vi "DB - [Execute].[Transaction].vi"(0 "connection reference":T12, 1 "DB.Schema.Table":string="SRTRS.Execute.TransactionResult", 2 "DB.Schema.Table 2\n(NA)":string, 3 "String ([RawDataFile] Filestream)":string, 4 "Transaction":T4, 5 "error in (no error)":errorcluster, 6 "DB Connection":T8={"Open"=TRUE, "Close"=TRUE}, 7 "Refnums":T7, 8 "DB - Execute Transaction":T6, 9 "[RawDataFileName]":string, 10 "[TransactionResult] v02":T5[](array[typedef]), 11 "DB Refnums II":T2, 12 "<Values>":string[](array[string])) -> (14 "connection reference":T12, 16 "1D Results":string[](array[string]), 18 "Transaction":T4, 19 "SUMMARY":errorcluster)   [LabVIEW 2013]
uses:
  <vilib>/addons/database/Connection.llb/Conn ObjectReference.ctl
  Controls/Setup - Part Details - Item Details.ctl
  Controls/Combo Box.ctl
  Controls/DB - Logon Info.ctl
  Controls/DB - OpenClose.ctl
  Controls/DB - Refnums.ctl
  Controls/DB - Execute Transaction Enum.ctl
  Controls/DB - [TransactionResult] Enum.ctl
  Controls/Transaction Cluster.ctl
  Controls/DB - Refnums II.ctl
  Controls/Execute - Info.ctl
  Controls/DB - [Execute].[Header] ColNames.ctl
  Controls/Global SRTRS.vi
  <vilib>/addons/database/Connection.llb/DB Tools Open Connec (String).vi
  <vilib>/addons/database/Connection.llb/Conn Execute.vi
  <vilib>/addons/database/Recordset.llb/Rec Fetch String Data (R).vi
  <vilib>/addons/database/Recordset.llb/Rec Destroy - Connection.vi
  <vilib>/addons/database/Recordset.llb/Rec Fetch Recordset Data (R).vi
  <vilib>/addons/database/NI_Database_API.lvlib
panel:
  in  "Equipment Details":i32(listbox)=-1
  in  "Info. (Execute Tab)":T1 caption="Info." {"Variant Allowed (Hold Temp)" format="%.1f"}
  in  "Results Output":cluster{"Output Set":T3, "Description":string}
  out "Close error out":errorcluster
  in  "MCListBox FHS Setup":i32(listbox)=-1 caption="Furnace Heating Sequence"
  out "Refnums error out":errorcluster={"status"=TRUE, "code"=1055, "source"="To More Specific Class in DB - Setup Item (Part Details).vi->Main.vi"}
  in  "Part Details":i32(listbox)=-1
  in  "MCListBox AWPS":i32(listbox)=-1 caption="Additional WPS/Ref MCListBox"
  in  "Logon":T9={"PlantID"="4070", "SystemID"="SRSB-2A", "UserID"="100001", "DomainID"="CCC", "LanguageID"="EN", "StationID"=""}
  in  "WPS Details Setup":T10={"WPS/Ref"="WPS5", "Rev"="1", "Hold Temperature"="100", "WPS Details Temperature Units"="°C", "Hold Time (HH:MM)"="1:00", "Inactive"=FALSE} caption="WPS Details"
  in  "Extra WPS":string caption="WPS"
  in  "Extra Rev":string caption="Rev."
  out "SQL 1":string
  in  "Item Details":T11={"Order No."="102", "Oper. No."="102", "Qty."=1, "NCR No."="102", "NCR Boolean"=FALSE, "Customer No."="102", "Customer Name"="Cust102", "Project"="Proj102", "Sales Order"="SO102", "Item No."="SOI102", "Material"="M102", "Revision"="1", "Material Description"="", "Serial No."="102", "UnitOfQty"="Pallet"} {"Qty." min=1 max=99}
  in  "Notes":string="Hello World"
  out "ms":u32
  out "SQL 2":string="USE [SRTRS]\n\nIF EXISTS(SELECT 1 from [Config].[Mapping]\nwhere [TransactionNo] = '<A>' )\n\nBEGIN\nDELETE FROM [MasterData].[Material]\nWHERE  [TransactionNo] = '<A>' \nEND\n\nINSERT INTO [Config].[Mapping]\n           ([TransactionNo]\n           ,[ItemNo]\n           ,[OrderNo]\n           ,[OperationNo]\n           ,[Qty]\n           ,[UnitOfQty]\n           ,[NCRIndicator]\n           ,[NCRNo]\n           ,[CustomerID]\n           ,[Customer]\n           ,[Project]\n           ,[SalesOrderNo]\n           ,[SalesOrderItemNo]\n           ,[MaterialNo]\n           ,[MaterialDesc]\n           ,[MaterialRev]\n           ,[SerialNos]\n           ,[Notes]\n           ,[TC01]  ,[TC02]  ,[TC03] ,[TC04] ,[TC05] ,[TC06] \n           ,[TC01Plot] ,[TC02Plot] ,[TC03Plot] ,[TC04Plot] ,[TC05Plot] ,[TC06Plot] \n           )\nVALUES (('' ,'1' ,'SOI101' ,'101' ,'101' ,'1' ,'EA' ,'FALSE' ,'101' ,'101' ,'Cust101' ,'Proj101' ,'SO101' ,'SOI101' ,'M101' ,'MD101' ,'1' ,'101' ,'' ,'1' ,'' ,'' ,'' ,'' ,'' ,'' ,'' ,'' ,'' ,'' ,'' ),('' ,'2' ,'SOI102' ,'102' ,'102' ,'1' ,'Pallet' ,'FALSE' ,'102' ,'102' ,'Cust102' ,'Proj102' ,'SO102' ,'SOI102' ,'M102' ,'2' ,'1' ,'102' ,'' ,'2' ,'' ,'' ,'' ,'' ,'' ,'' ,'' ,'' ,'' ,'' ,'' ))\n\n-- SELECT SCOPE_IDENTITY()"
  out "Connection Information":T13={"Connection "="SQL Server 32bit HPEnvy", "Username"="admin", "Password"="admin123"}
  # "Column Hdrs[] are Important \nMust match with SRTRS Main.vi"
  # "Min"
  # "Min"
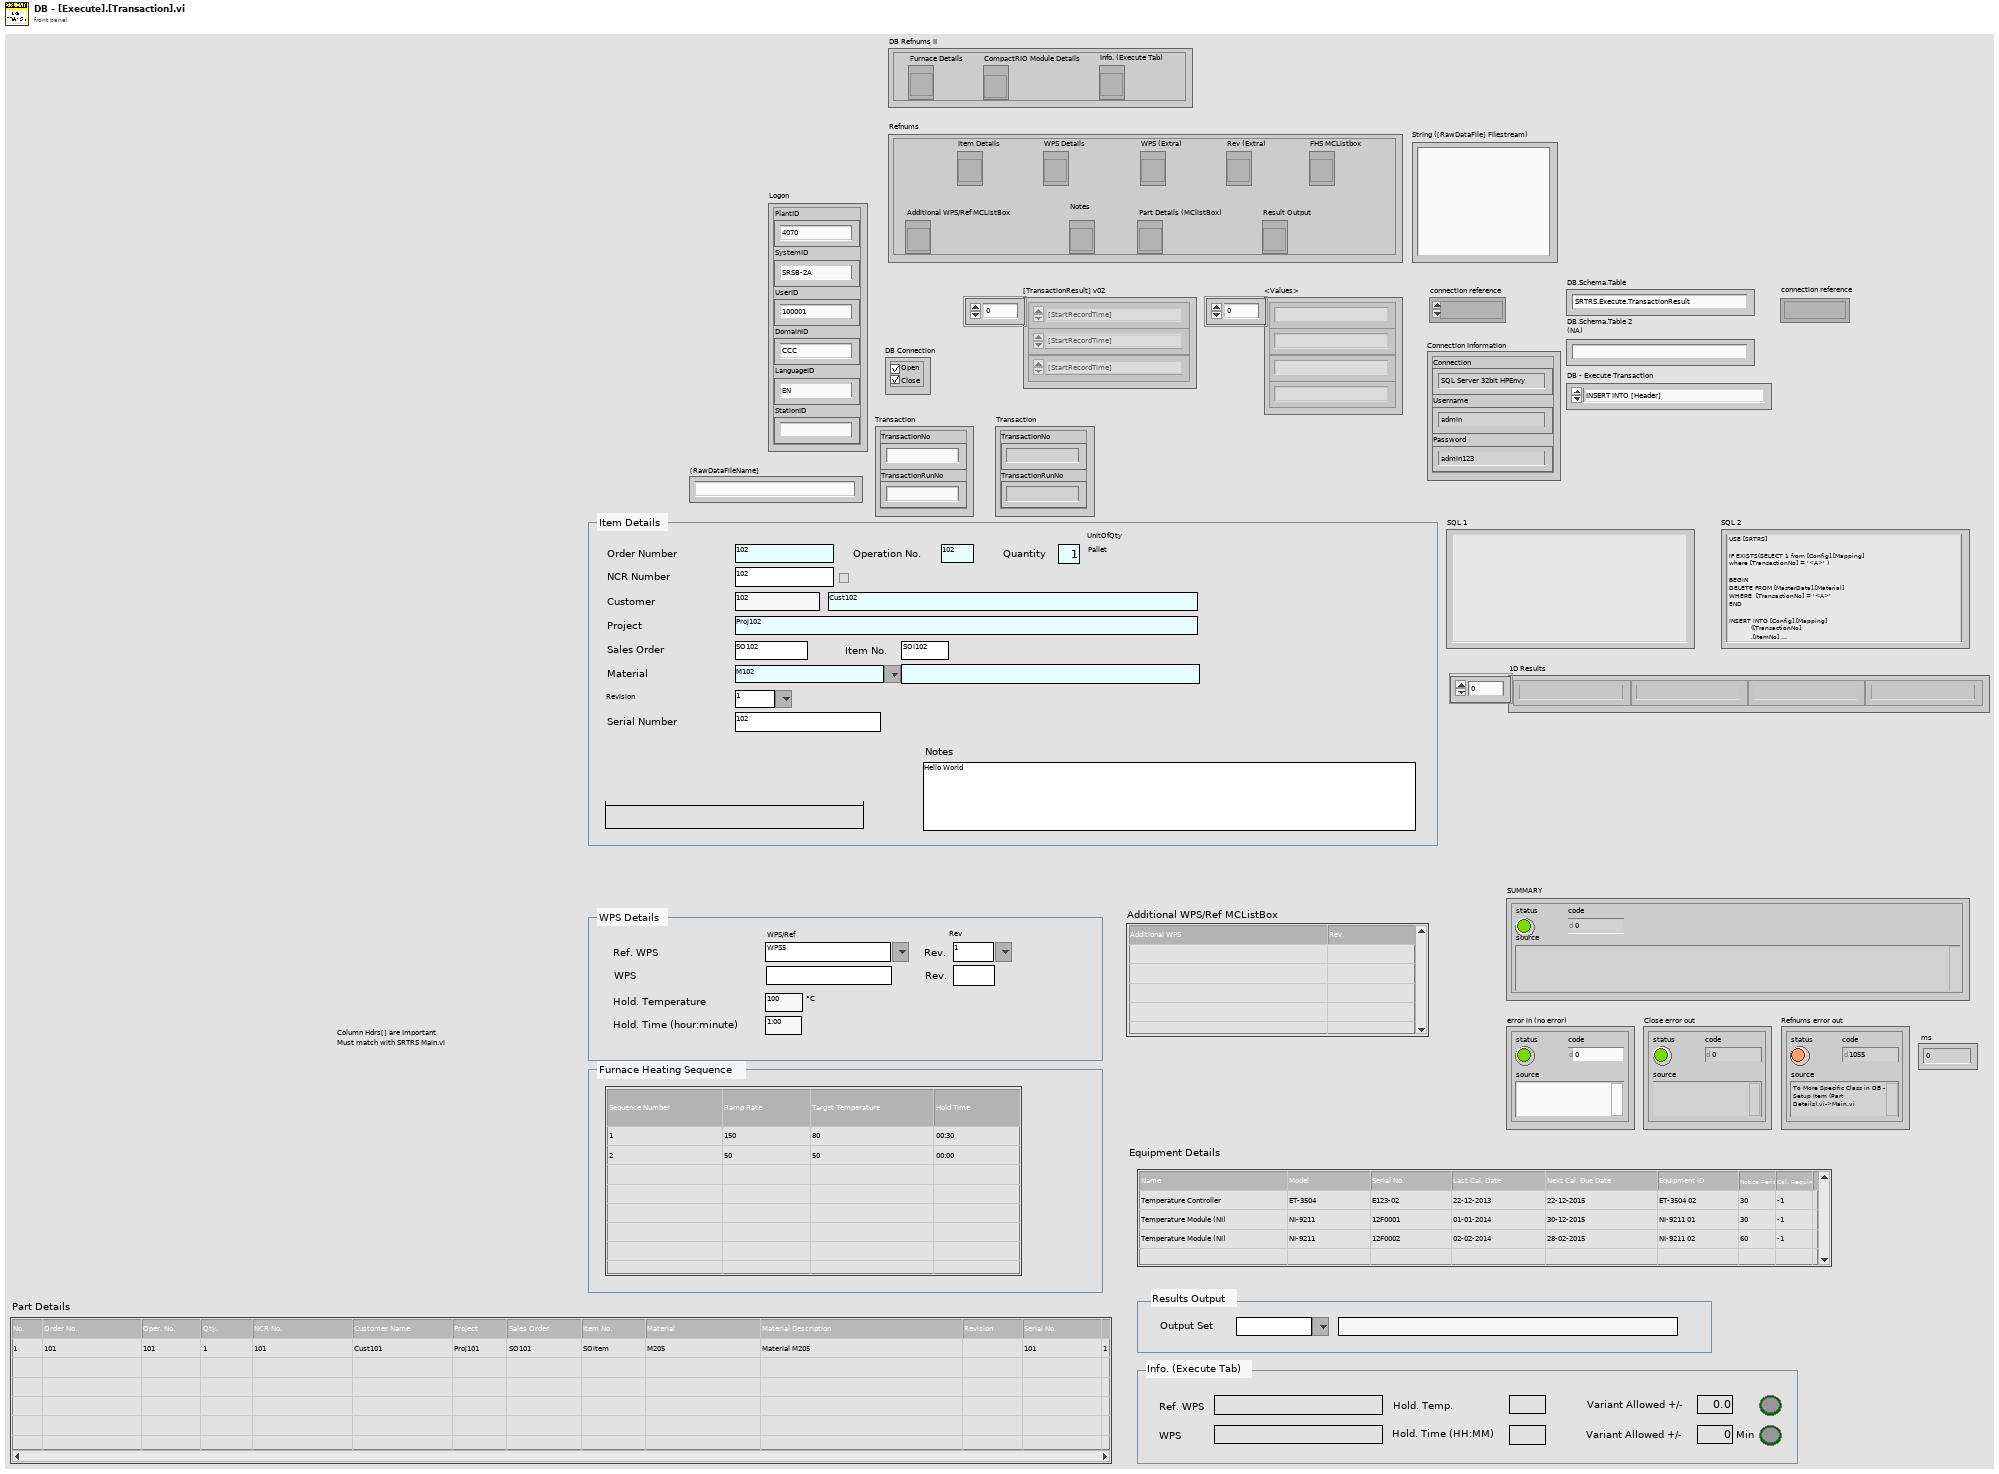
[diagram p1: front panel]
types:
  T1 = typedef "Execute - Info.ctl" = cluster{"Ref WPS":string, "Hold. Temp.":string, "Info. Temperature Units":string, "Variant Allowed (Hold Temp)":dbl, "Info. Temperature Units 2":string, "Variant Allowed (Hold Temp)":bool, "Hold. Time (hour:minute)":string, "Variant Allowed (Hold Time)":dbl, "Variant Allowed (Hold Time)":bool, "WPS":string}
  T2 = typedef "DB - Refnums II.ctl" = cluster{"Furnace Details":refnum<vi>, "CompactRIO Module Details":refnum<vi>, "Info. (Execute Tab)":refnum<vi>}
  T3 = typedef "Combo Box.ctl" = string
  T4 = typedef "Transaction Cluster.ctl" = cluster{"TransactionNo":string, "TransactionRunNo":string}
  T5 = typedef "DB - [TransactionResult] Enum.ctl" = enum16{"[StartRecordTime]", "[StartRecordTemp]", "[MaxRecordedTemp]", "[MaxRecordedTempTime]", "[MinRecordedTemp]", "[MinRecordedTempTime]", "[EndRecordTemp]", "[EndRecordTime]", "[RecordedMinutes]", "[StartHoldTime]", "[StartHoldTemp]", "[HoldTimeMaxTemp]", "[HoldTimeMaxTempTime]", "[HoldTimeMinTemp]", "[HoldTimeMinTempTime]", "[EndHoldTime]", "[EndHoldTemp]", "[HoldDurationMinutes]", "[TempDiffDuringHold]", "[UnitOfTemperature]", "[PerformedBy]", "[PerformedOn]", "[IsTempWithinTol]", "[IsTimeWithinTol]", "[HoldTimePercentage]", "[ProcessStatus]", "[OverallStatus]", "[SequenceStatus]", "[Parameter1]", "[Parameter2]", "[Parameter3]", "[Parameter4]", "[Parameter5]", "[Parameter6]", "[Parameter7]", "[Parameter8]", "[Parameter9]", "[Parameter10]", "[Parameter11]", "[Parameter12]", "[Result]", "[RawDataFile]", "[RawDataFilePath]", "[RawDataFileName]", "[OutputSetId]", "[SavedBy]", "[SavedOn]", "[Inactive]"}
  T6 = typedef "DB - Execute Transaction Enum.ctl" = enum16{"INSERT INTO [Header]", "INSERT INTO [TransactionResult]", "INSERT INTO [ProcedureItem]", "INSERT/UPDATE [Execute].[Active]", "SELECT [Execute].[Active]", "UPDATE [TransactionResult]", "UPDATE FILESTREAM", "SELECT [TransactionResult]", "SELECT [TransactionNo],[TransactionRunNo]"}
  T7 = typedef "DB - Refnums.ctl" = cluster{"Item Details":refnum<vi>, "WPS Details":refnum<vi>, "WPS (Extra)":refnum<vi>, "Rev (Extra) ":refnum<vi>, "FHS MCListbox":refnum<vi>, "Additional WPS/Ref MCListBox":refnum<vi>, "Notes":refnum<vi>, "Part Details (MClistBox)":refnum<vi>, "Result Output":refnum<vi>}
  T8 = typedef "DB - OpenClose.ctl" = cluster{"Open":bool, "Close":bool}
  T9 = typedef "DB - Logon Info.ctl" = cluster{"PlantID":string, "SystemID":string, "UserID":string, "DomainID":string, "LanguageID":string, "StationID":string}
  T10 = cluster{"WPS/Ref":T3, "Rev":T3, "Hold Temperature":string, "WPS Details Temperature Units":string, "Hold Time (HH:MM)":string, "Inactive":bool}
  T11 = typedef "Setup - Part Details - Item Details.ctl" = cluster{"Order No.":string, "Oper. No.":string, "Qty.":i32, "NCR No.":string, "NCR Boolean":bool, "Customer No.":string, "Customer Name":string, "Project":string, "Sales Order":string, "Item No.":string, "Material":string, "Revision":string, "Material Description":string, "Serial No.":string, "UnitOfQty":string}
  T12 = typedef "NI_Database_API.lvlib/Conn ObjectReference.ctl" = refnum<k1>
  T13 = cluster{"Connection ":string, "Username":string, "Password":string}
  T14 = typedef "Enum - InteractiveMode-SubVIMode.ctl" = enum16{"Interactive", "subVI Mode"}
  T15 = typedef "Connection Information Cluster.ctl" = cluster{"Connection ":string, "Username":string, "Password":string}
  T16 = typedef "DB - DB.Schema.Table.ctl" = cluster{"DB":string, "Schema":string, "Table":string}
  T17 = typedef "DB - [Execute].[Header] ColNames.ctl" = enum16{"[SystemId]", "[PlantId]", "[StationId]", "[ProcedureNo]", "[ProcedureRev]", "[WpsNo]", "[WpsRev]", "[HoldTemperature]", "[UnitOfTemperature]", "[HoldTime]", "[OutputSetId]", "[AdditionalProcs]", "[Equipment1Id]", "[Equipment2Id]", "[Equipment3Id]", "[Equipment4Id]", "[Equipment5Id]", "[Equipment6Id]", "[Equipment7Id]", "[Equipment8Id]", "[Equipment9Id]", "[Equipment10Id]", "[PermittedTempDiff]", "[PermittedTimeDiff]", "[Notes]", "[LastSavedBy]", "[LastSavedOn]", "[Indicator1]", "[Indicator2]", "[Remark1]", "[Remark2]", "[Remark3]", "[Remark4]", "[Inactive]"}
  T18 = typedef "NI_Database_API.lvlib/Rec ObjectReference.ctl" = refnum<k1>
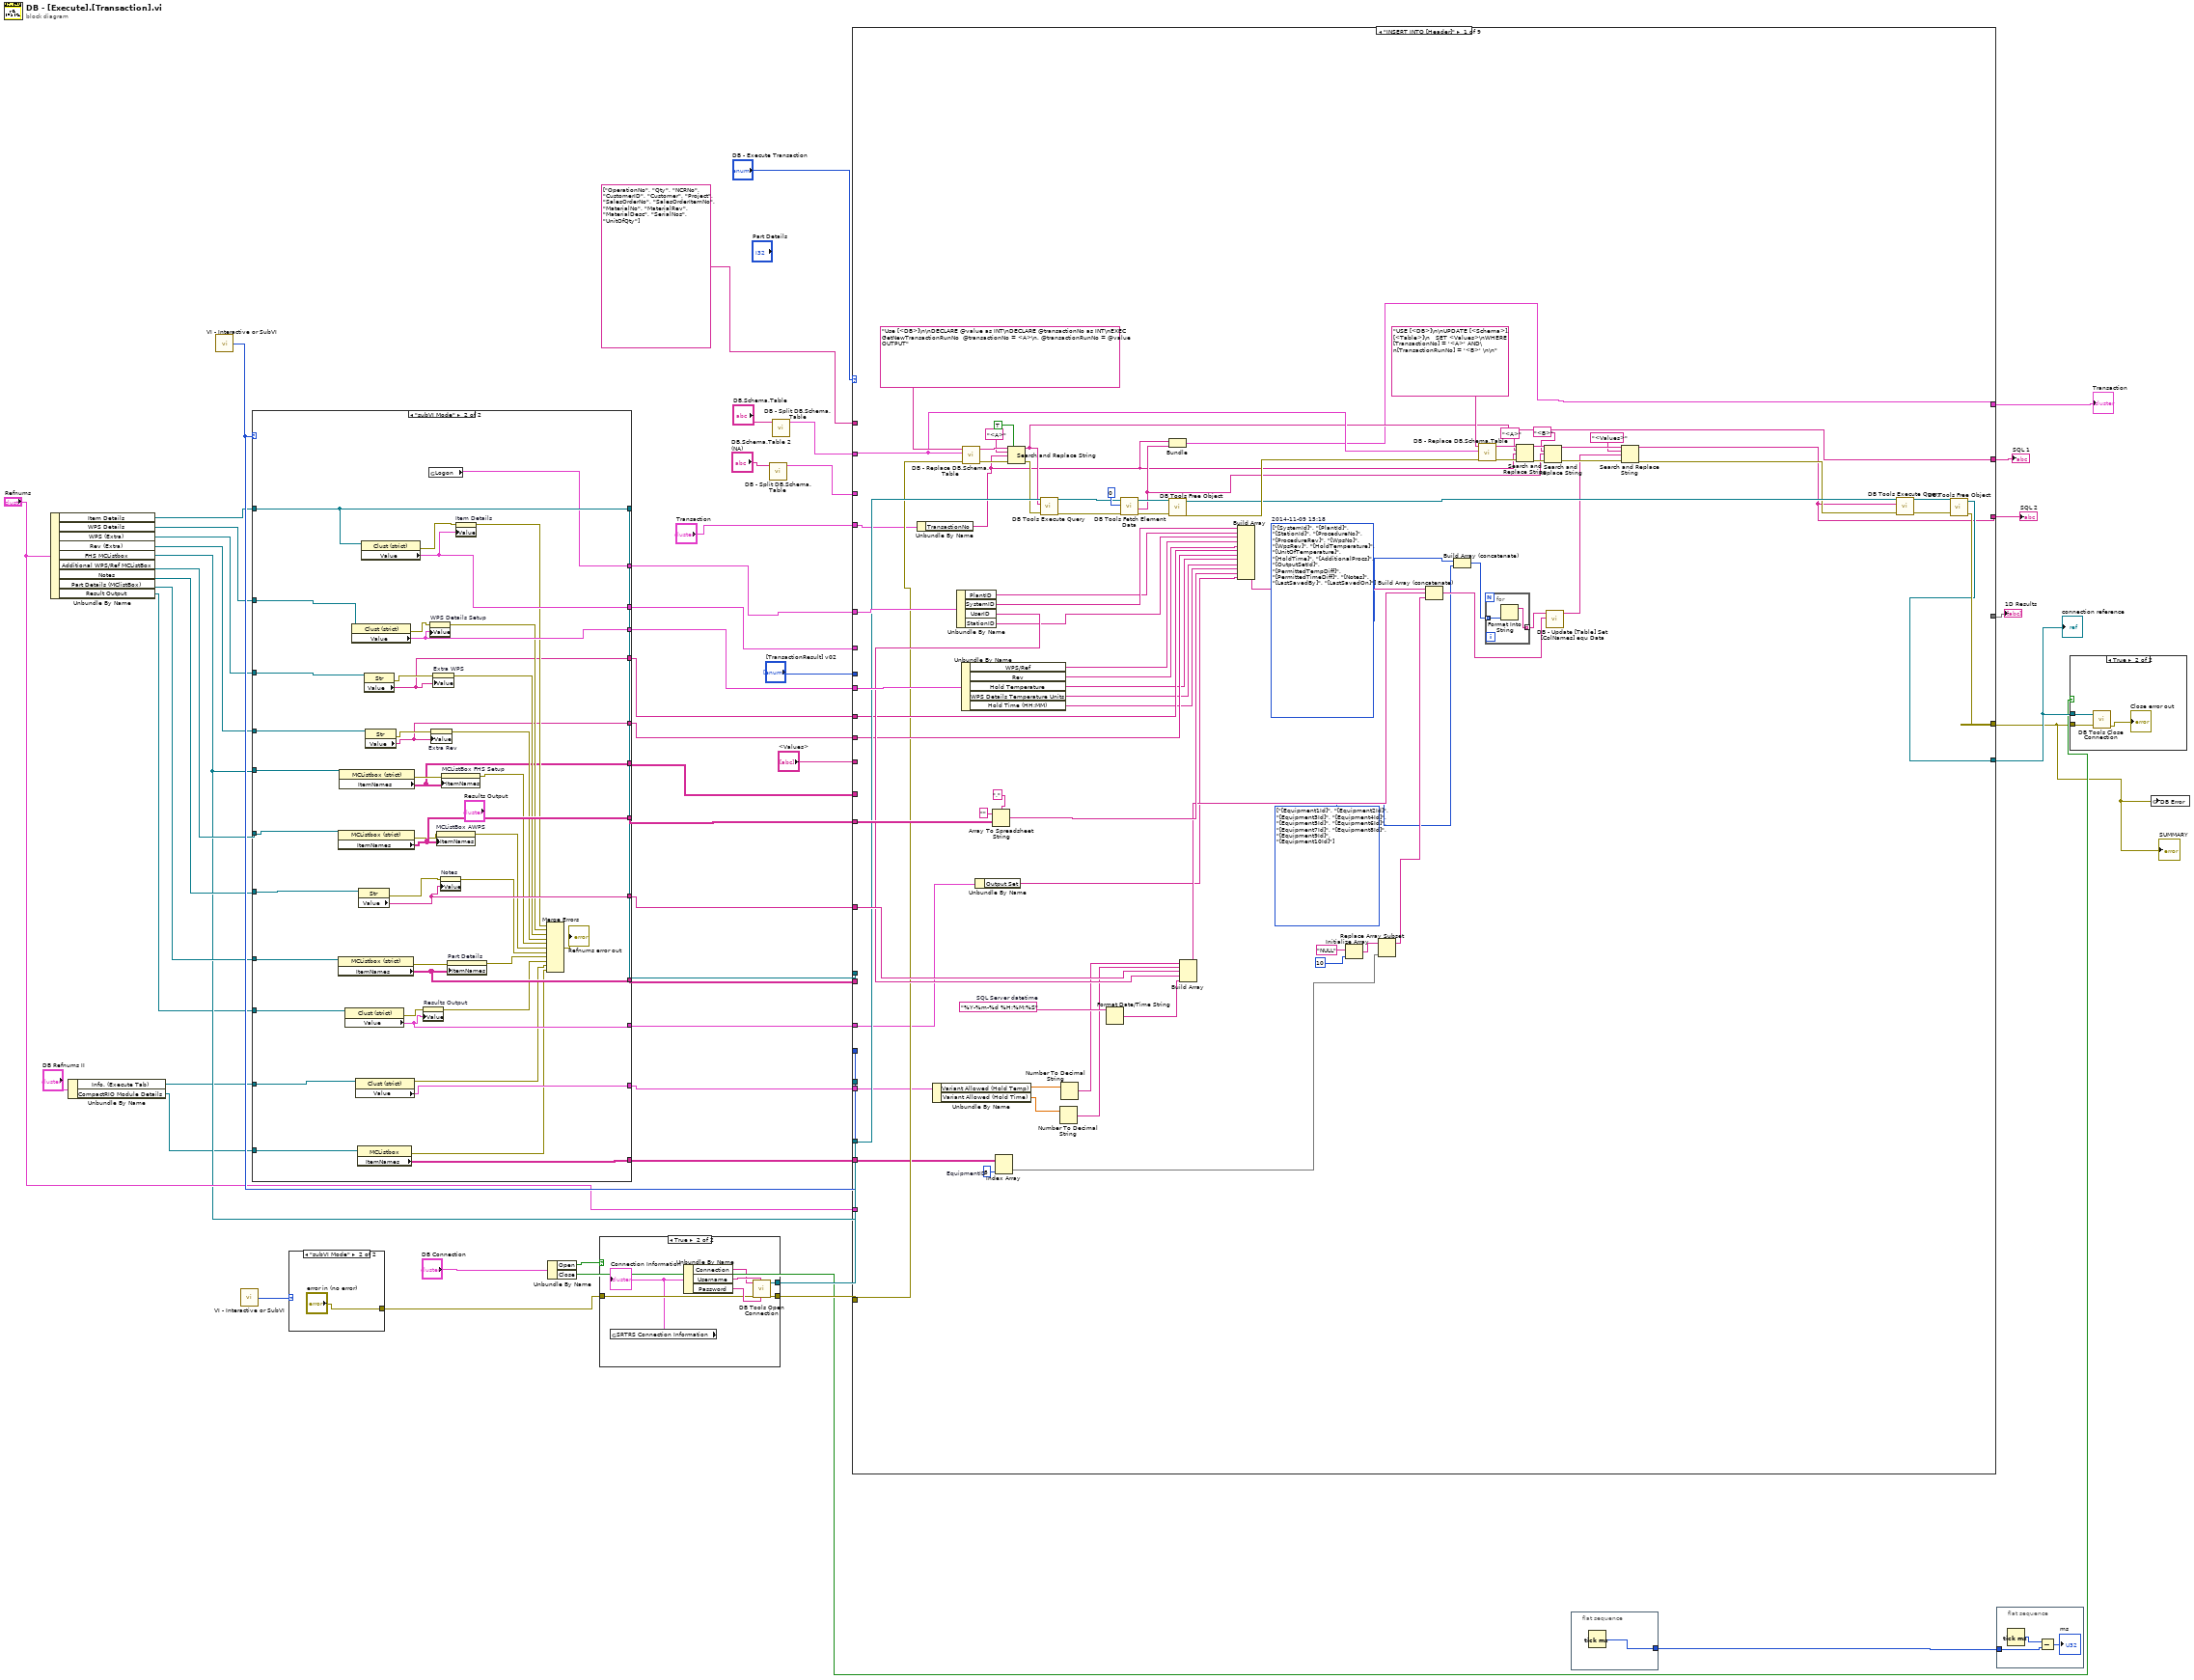
[diagram p0: block diagram]
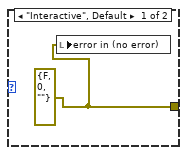
[diagram p2: hidden frame]
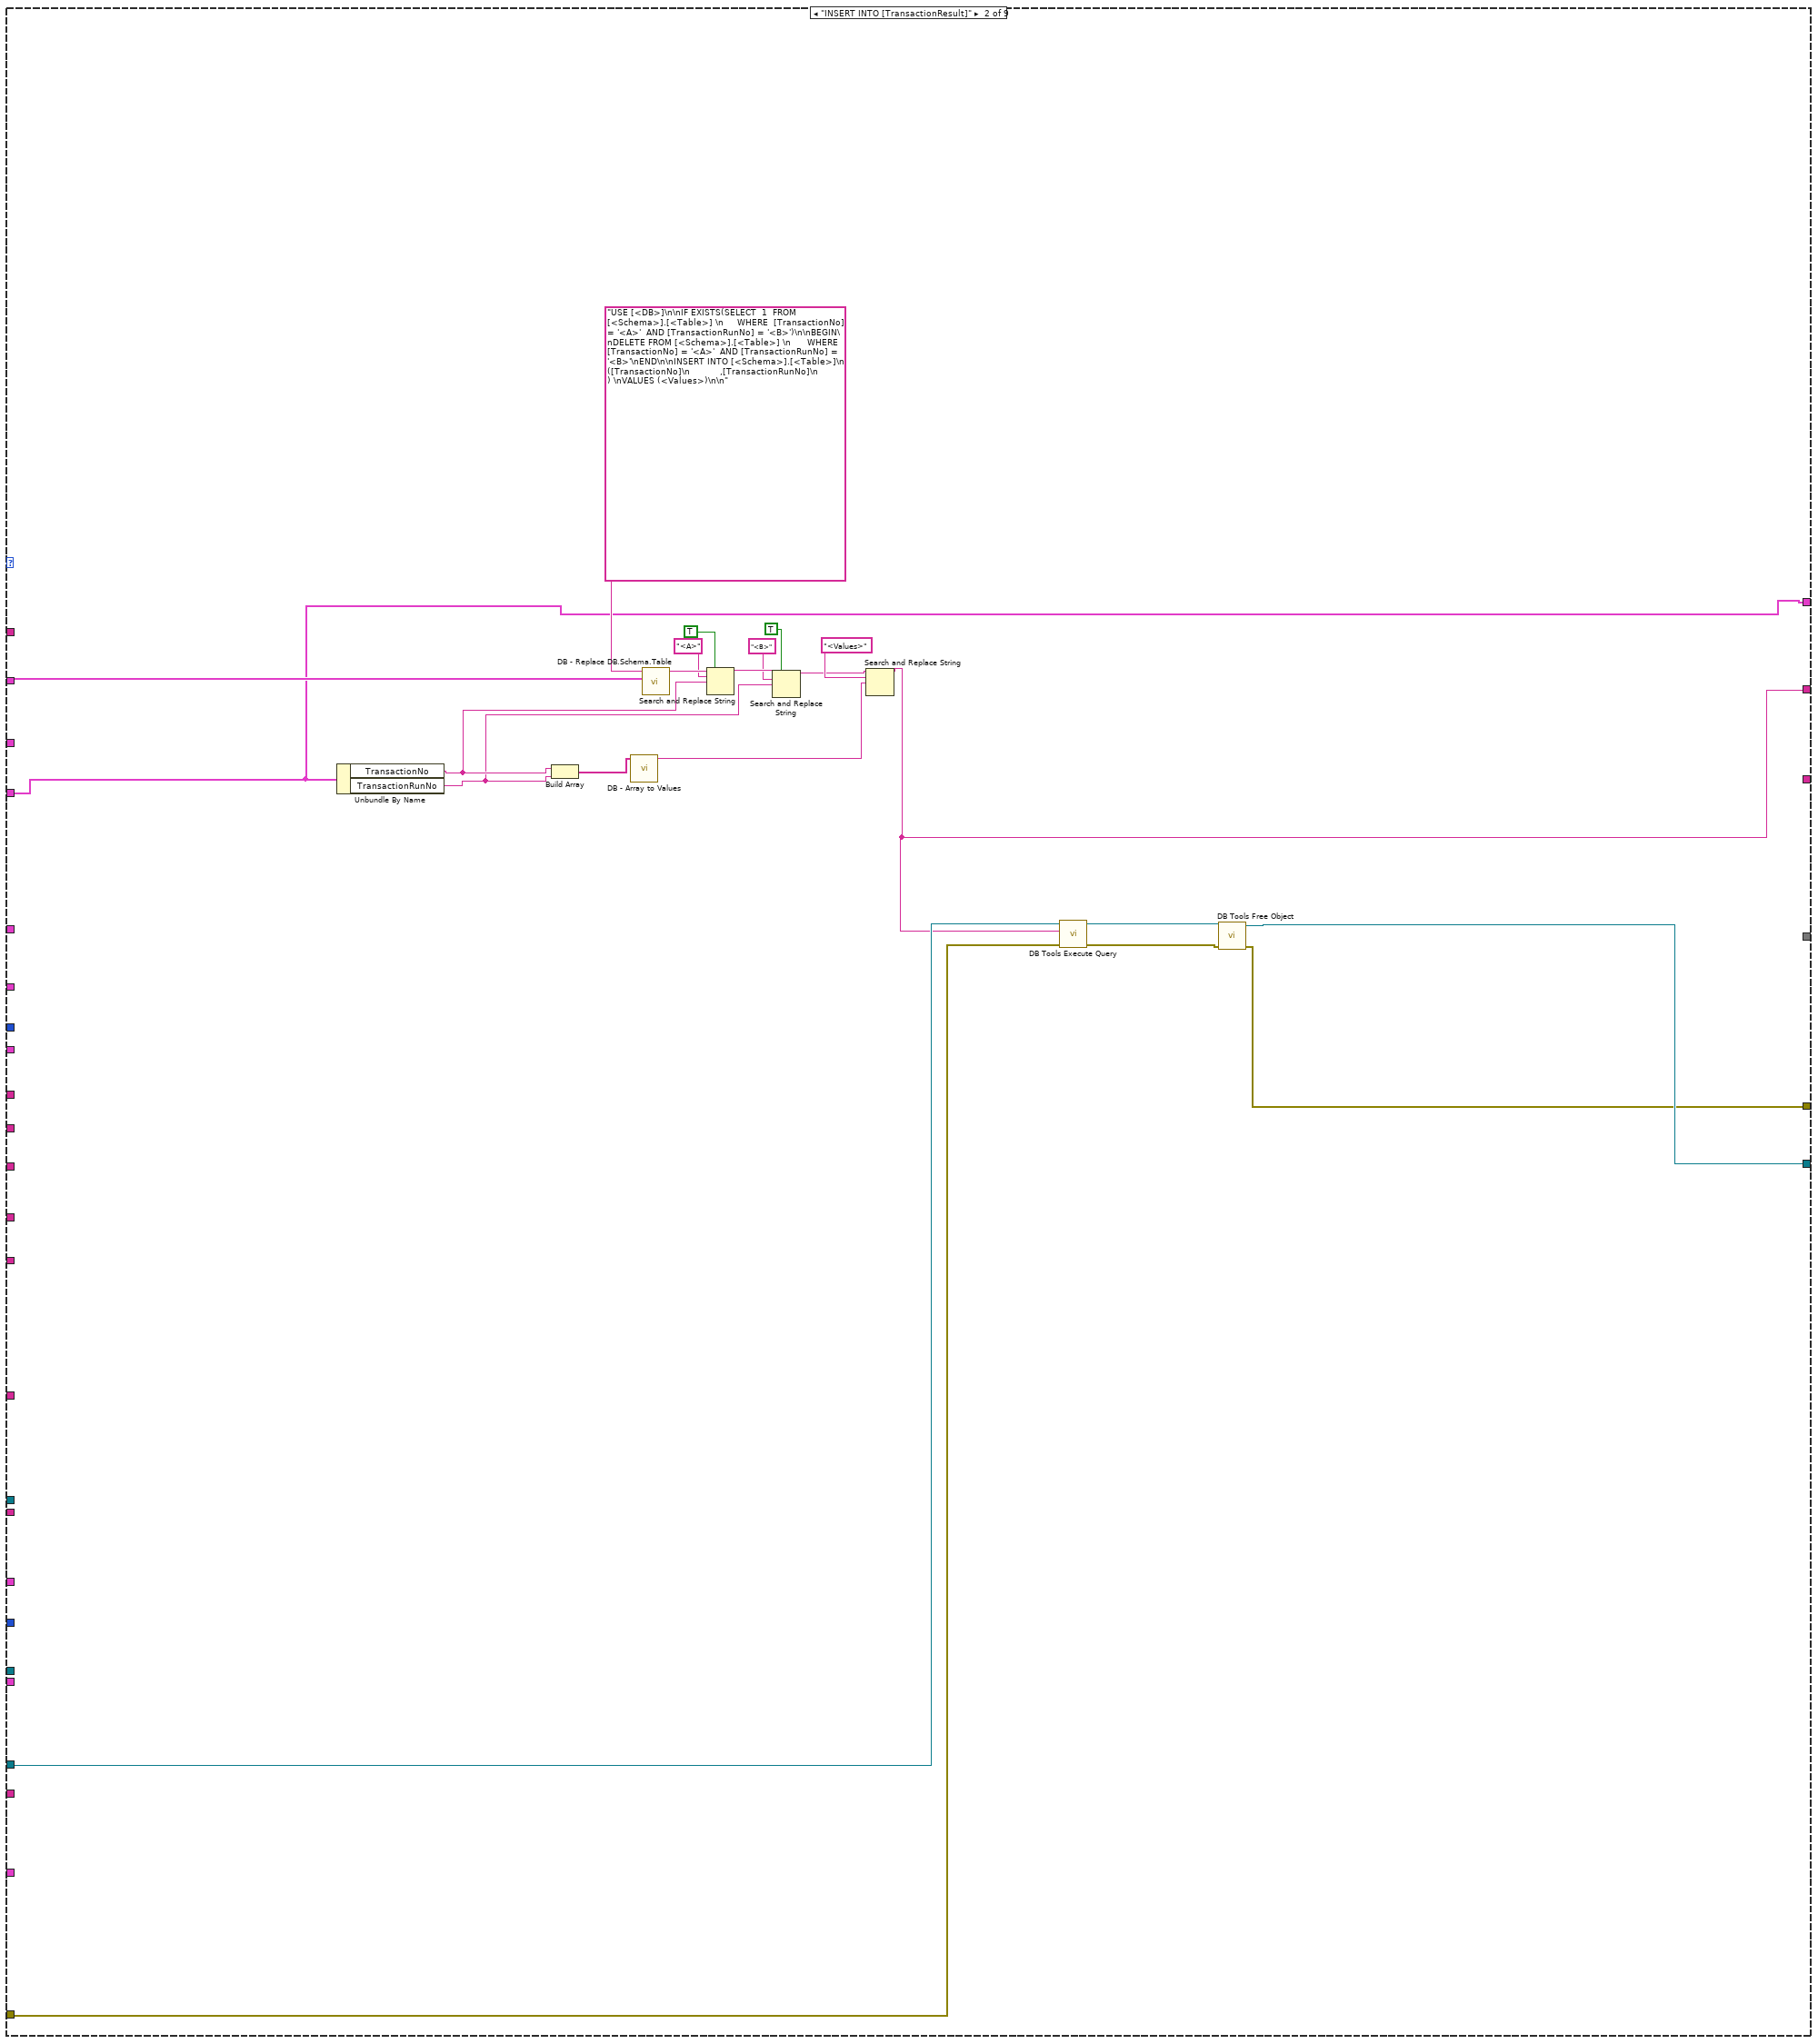
[diagram p3: hidden frame]
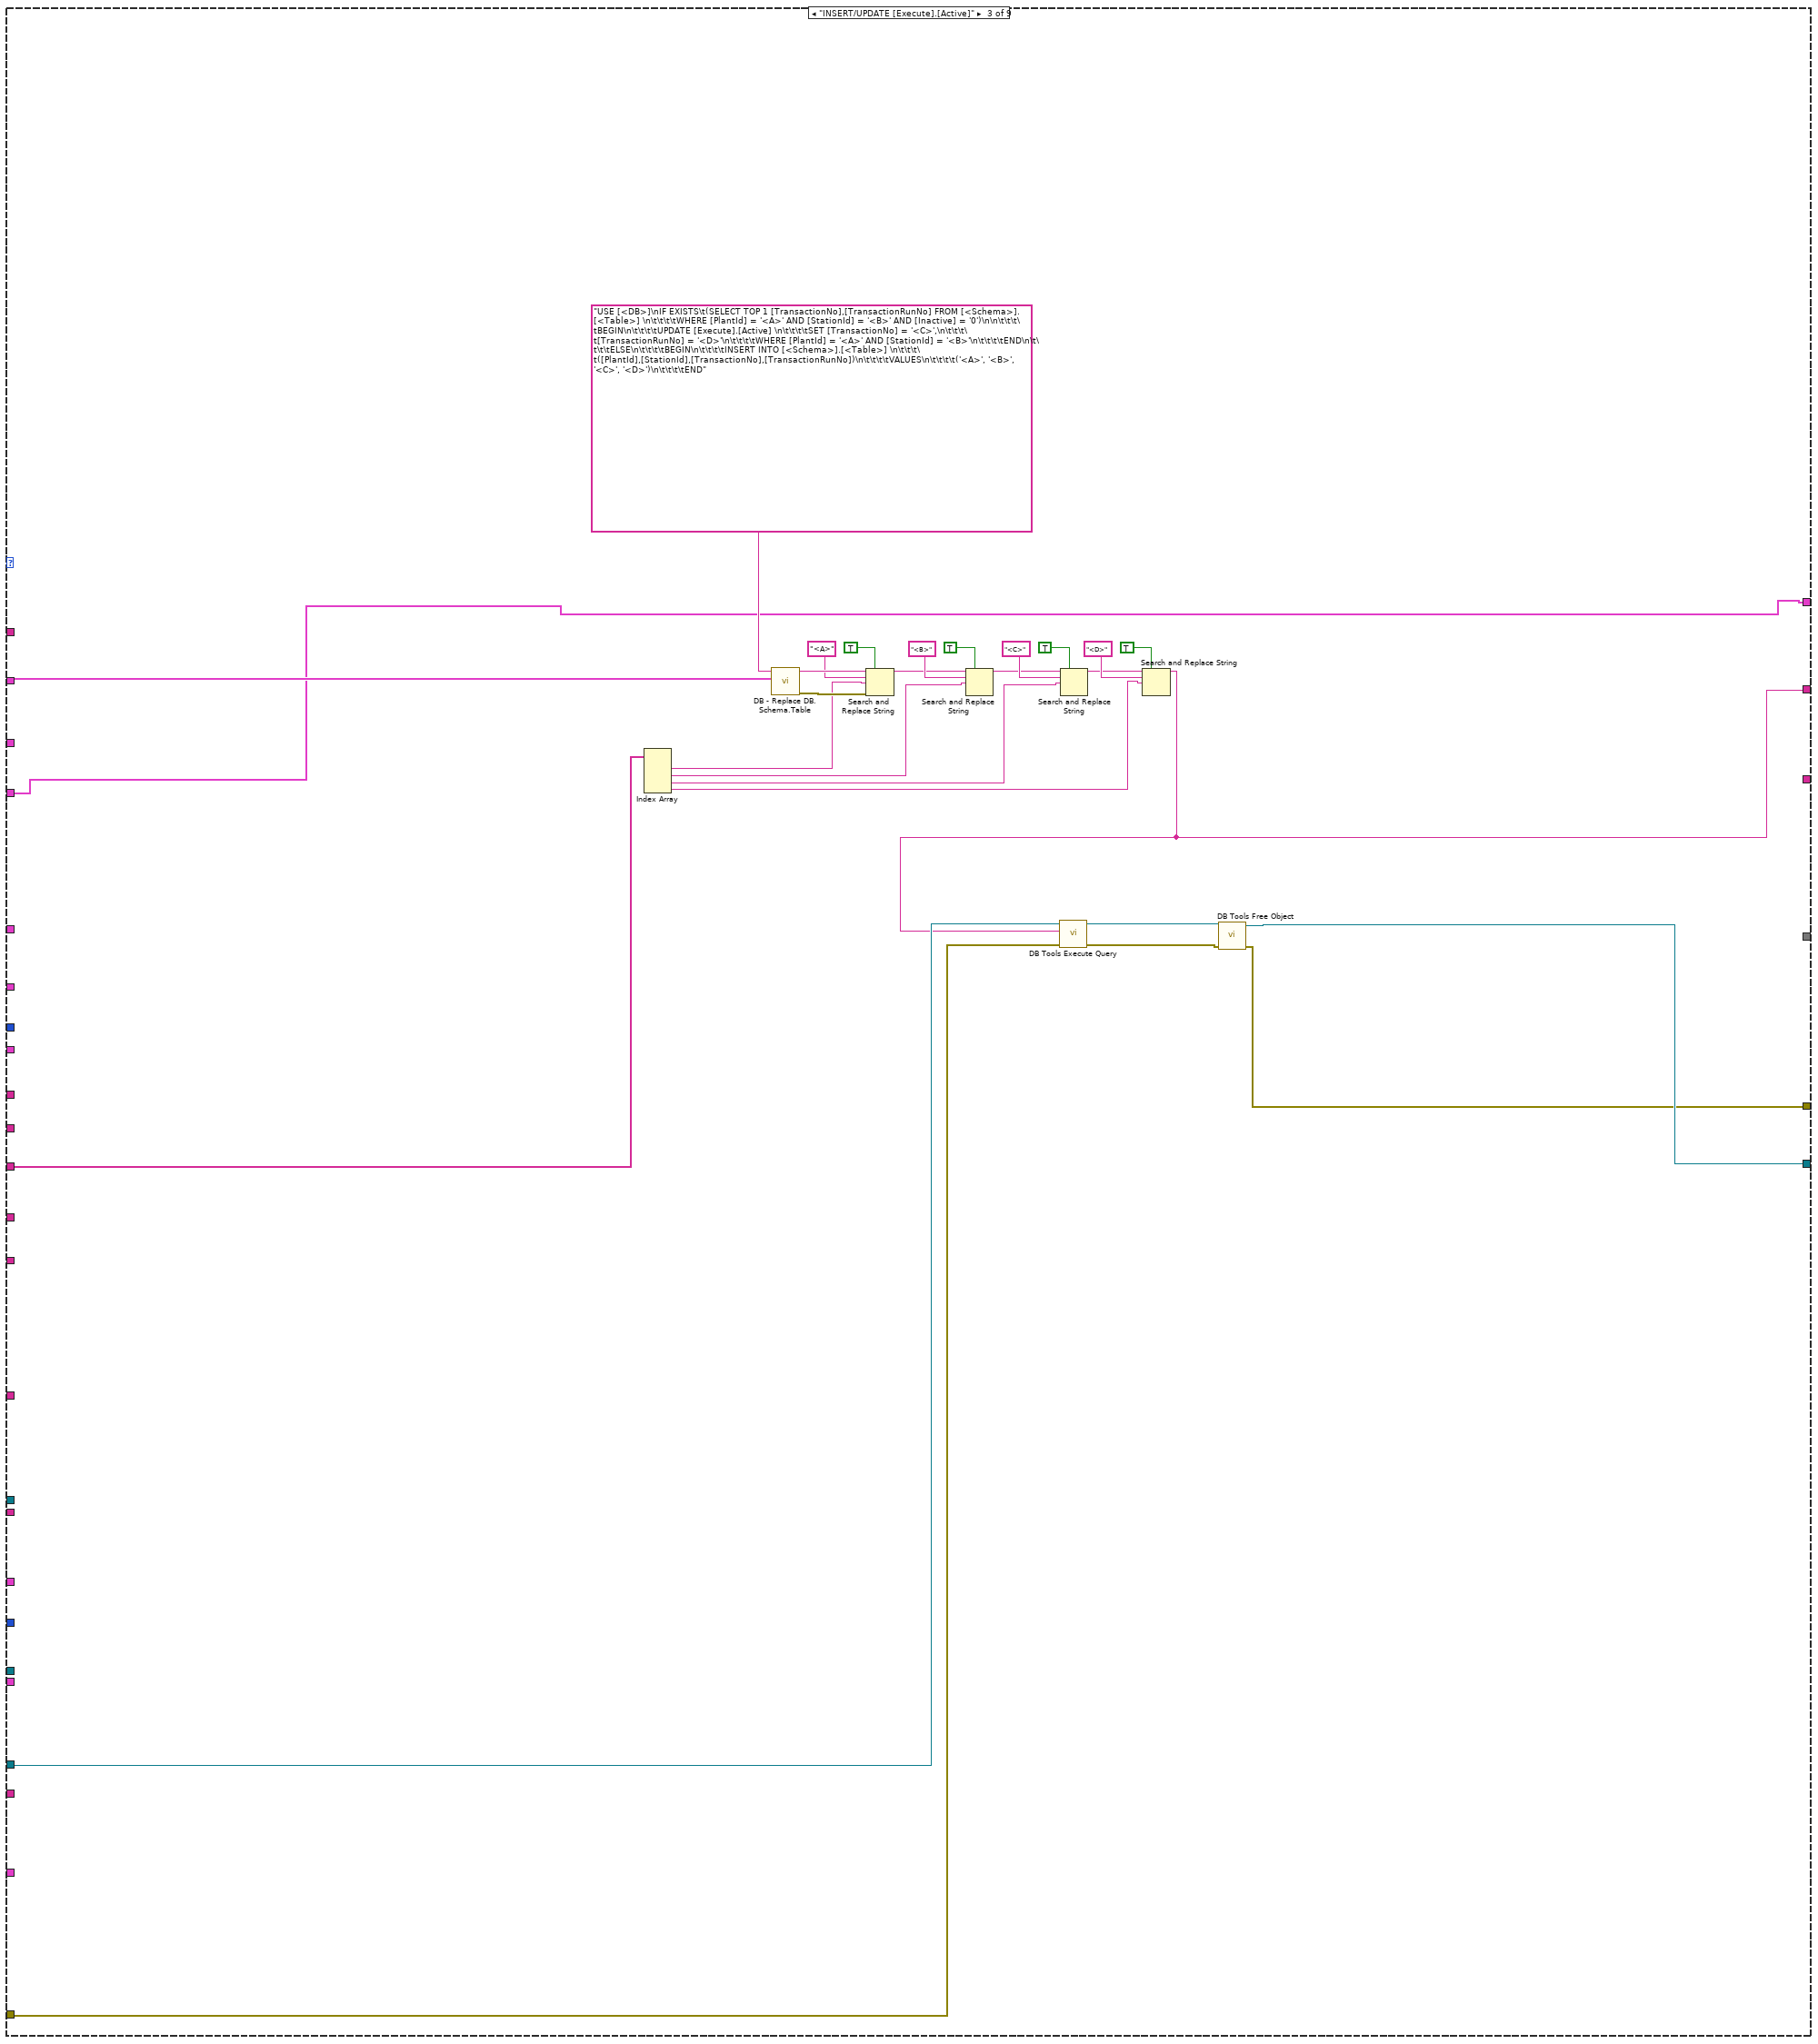
[diagram p4: hidden frame]
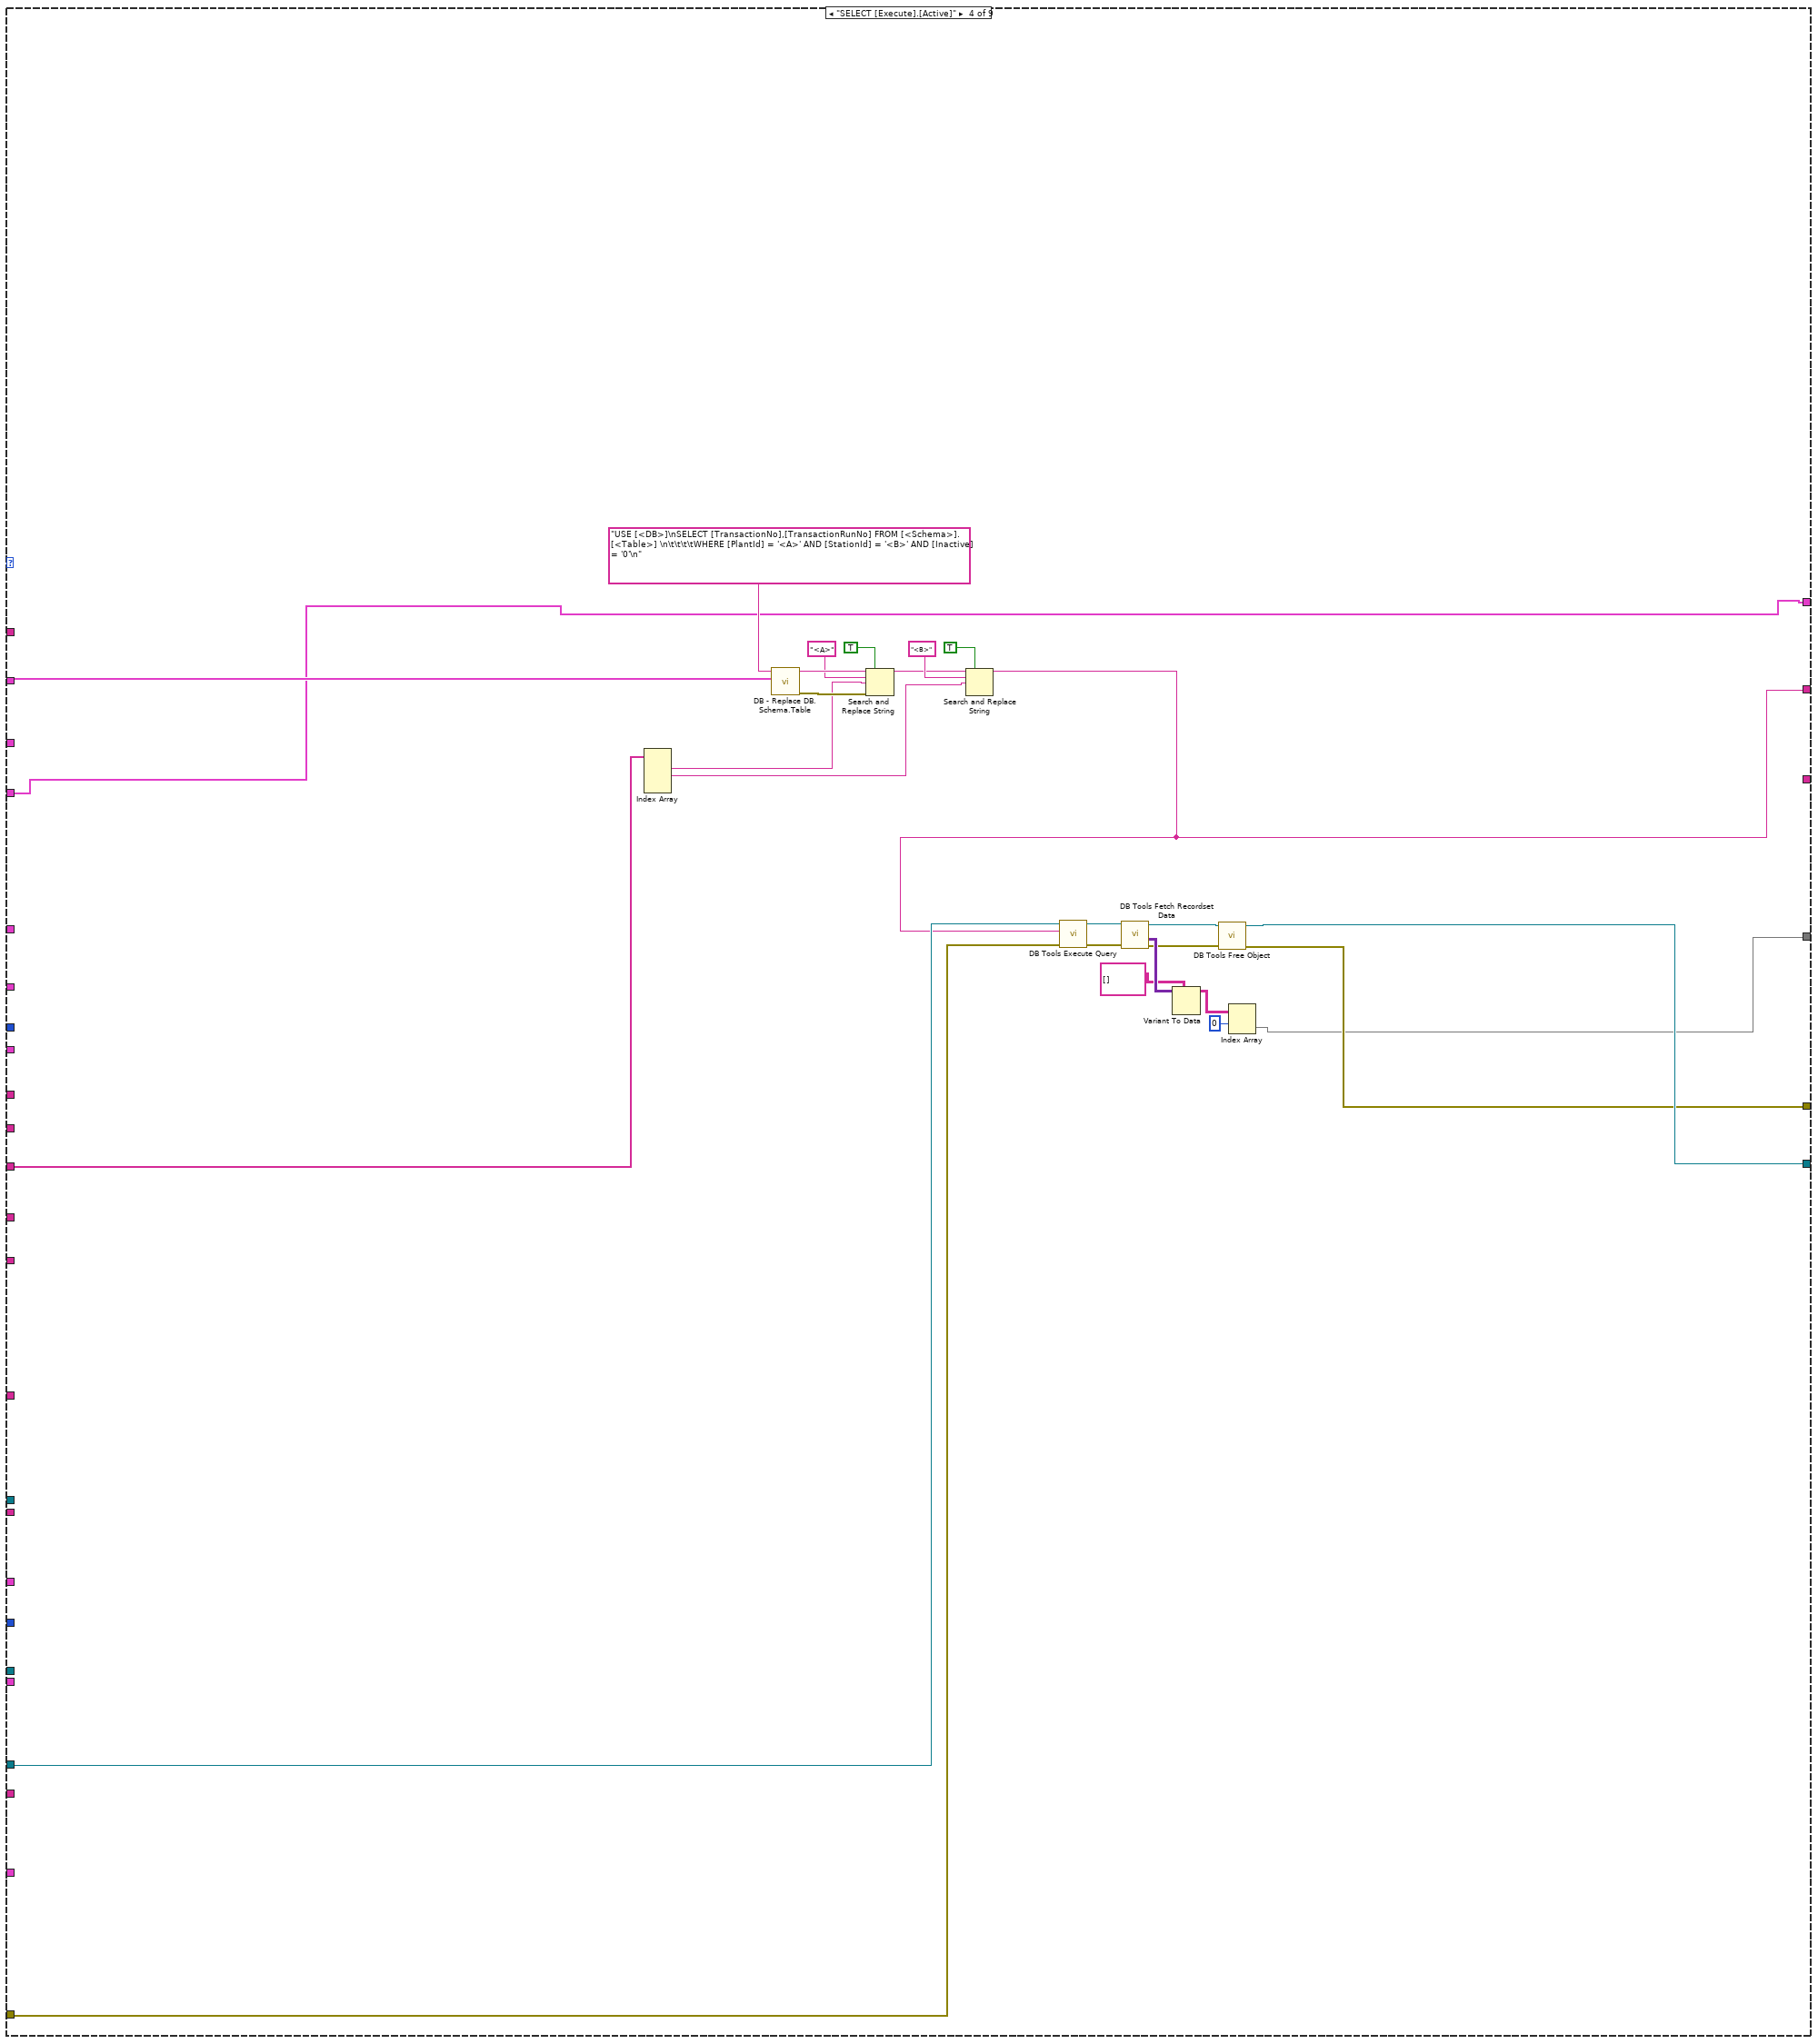
[diagram p5: hidden frame]
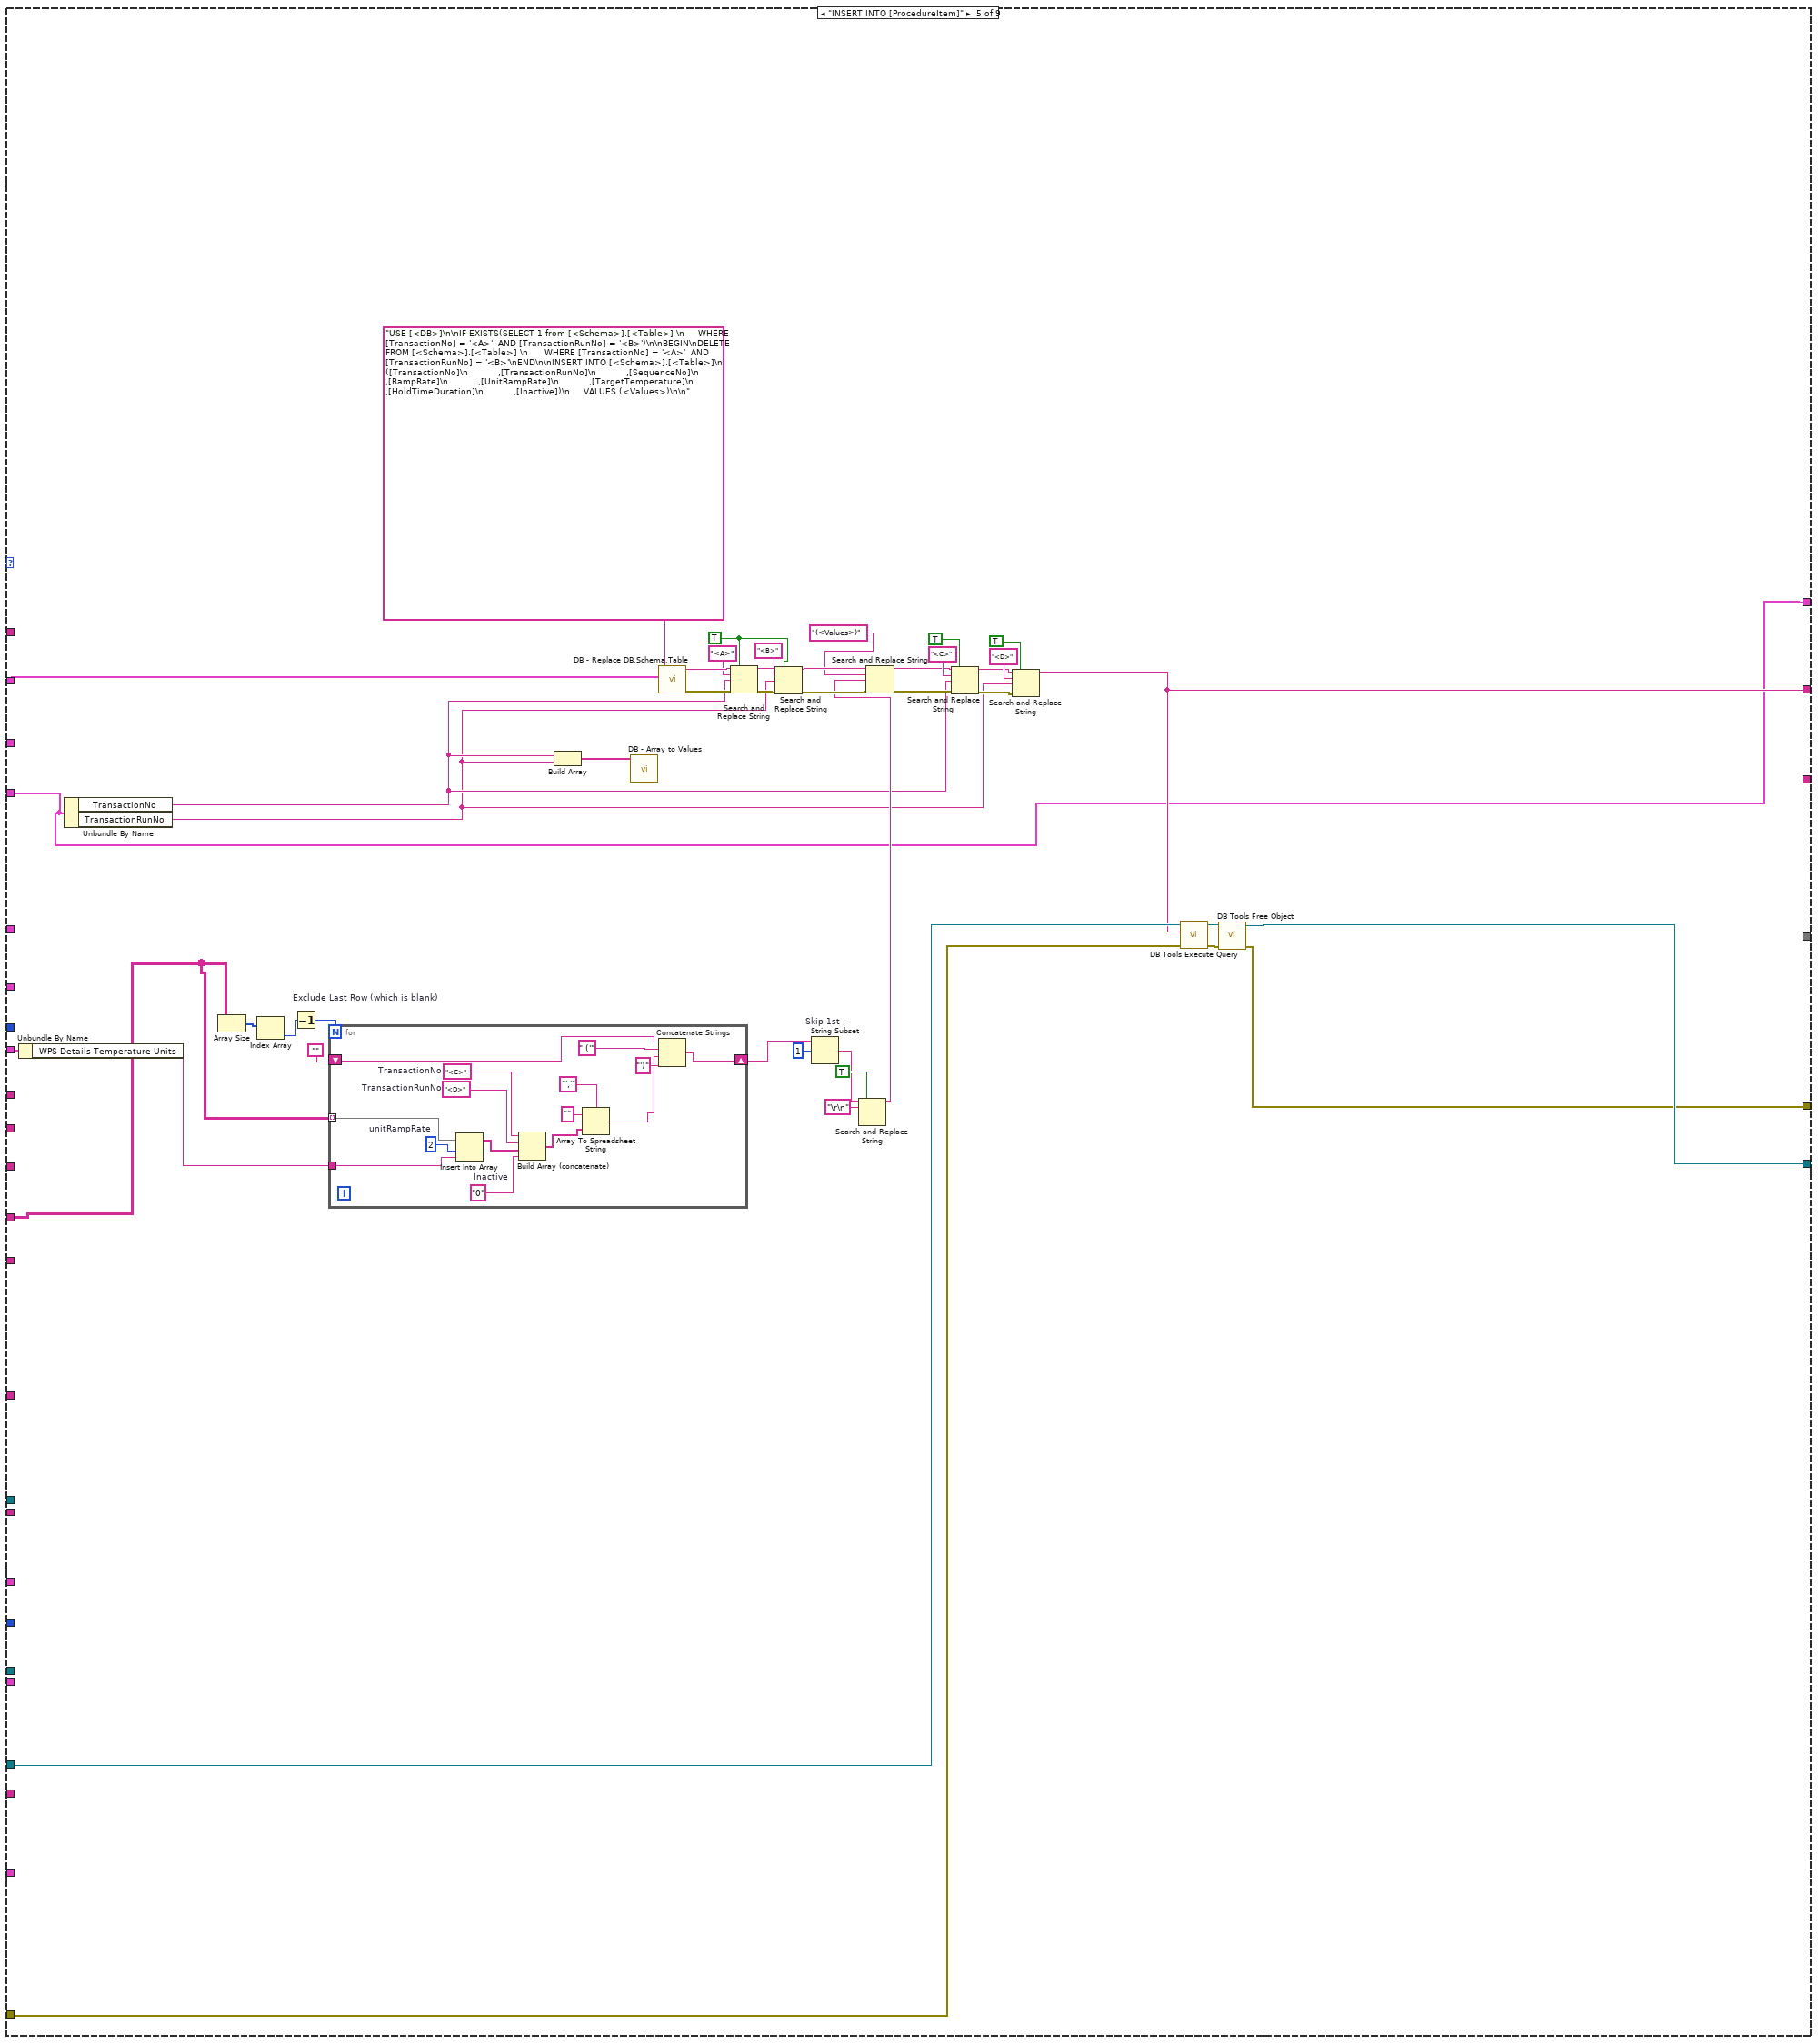
[diagram p6: hidden frame]
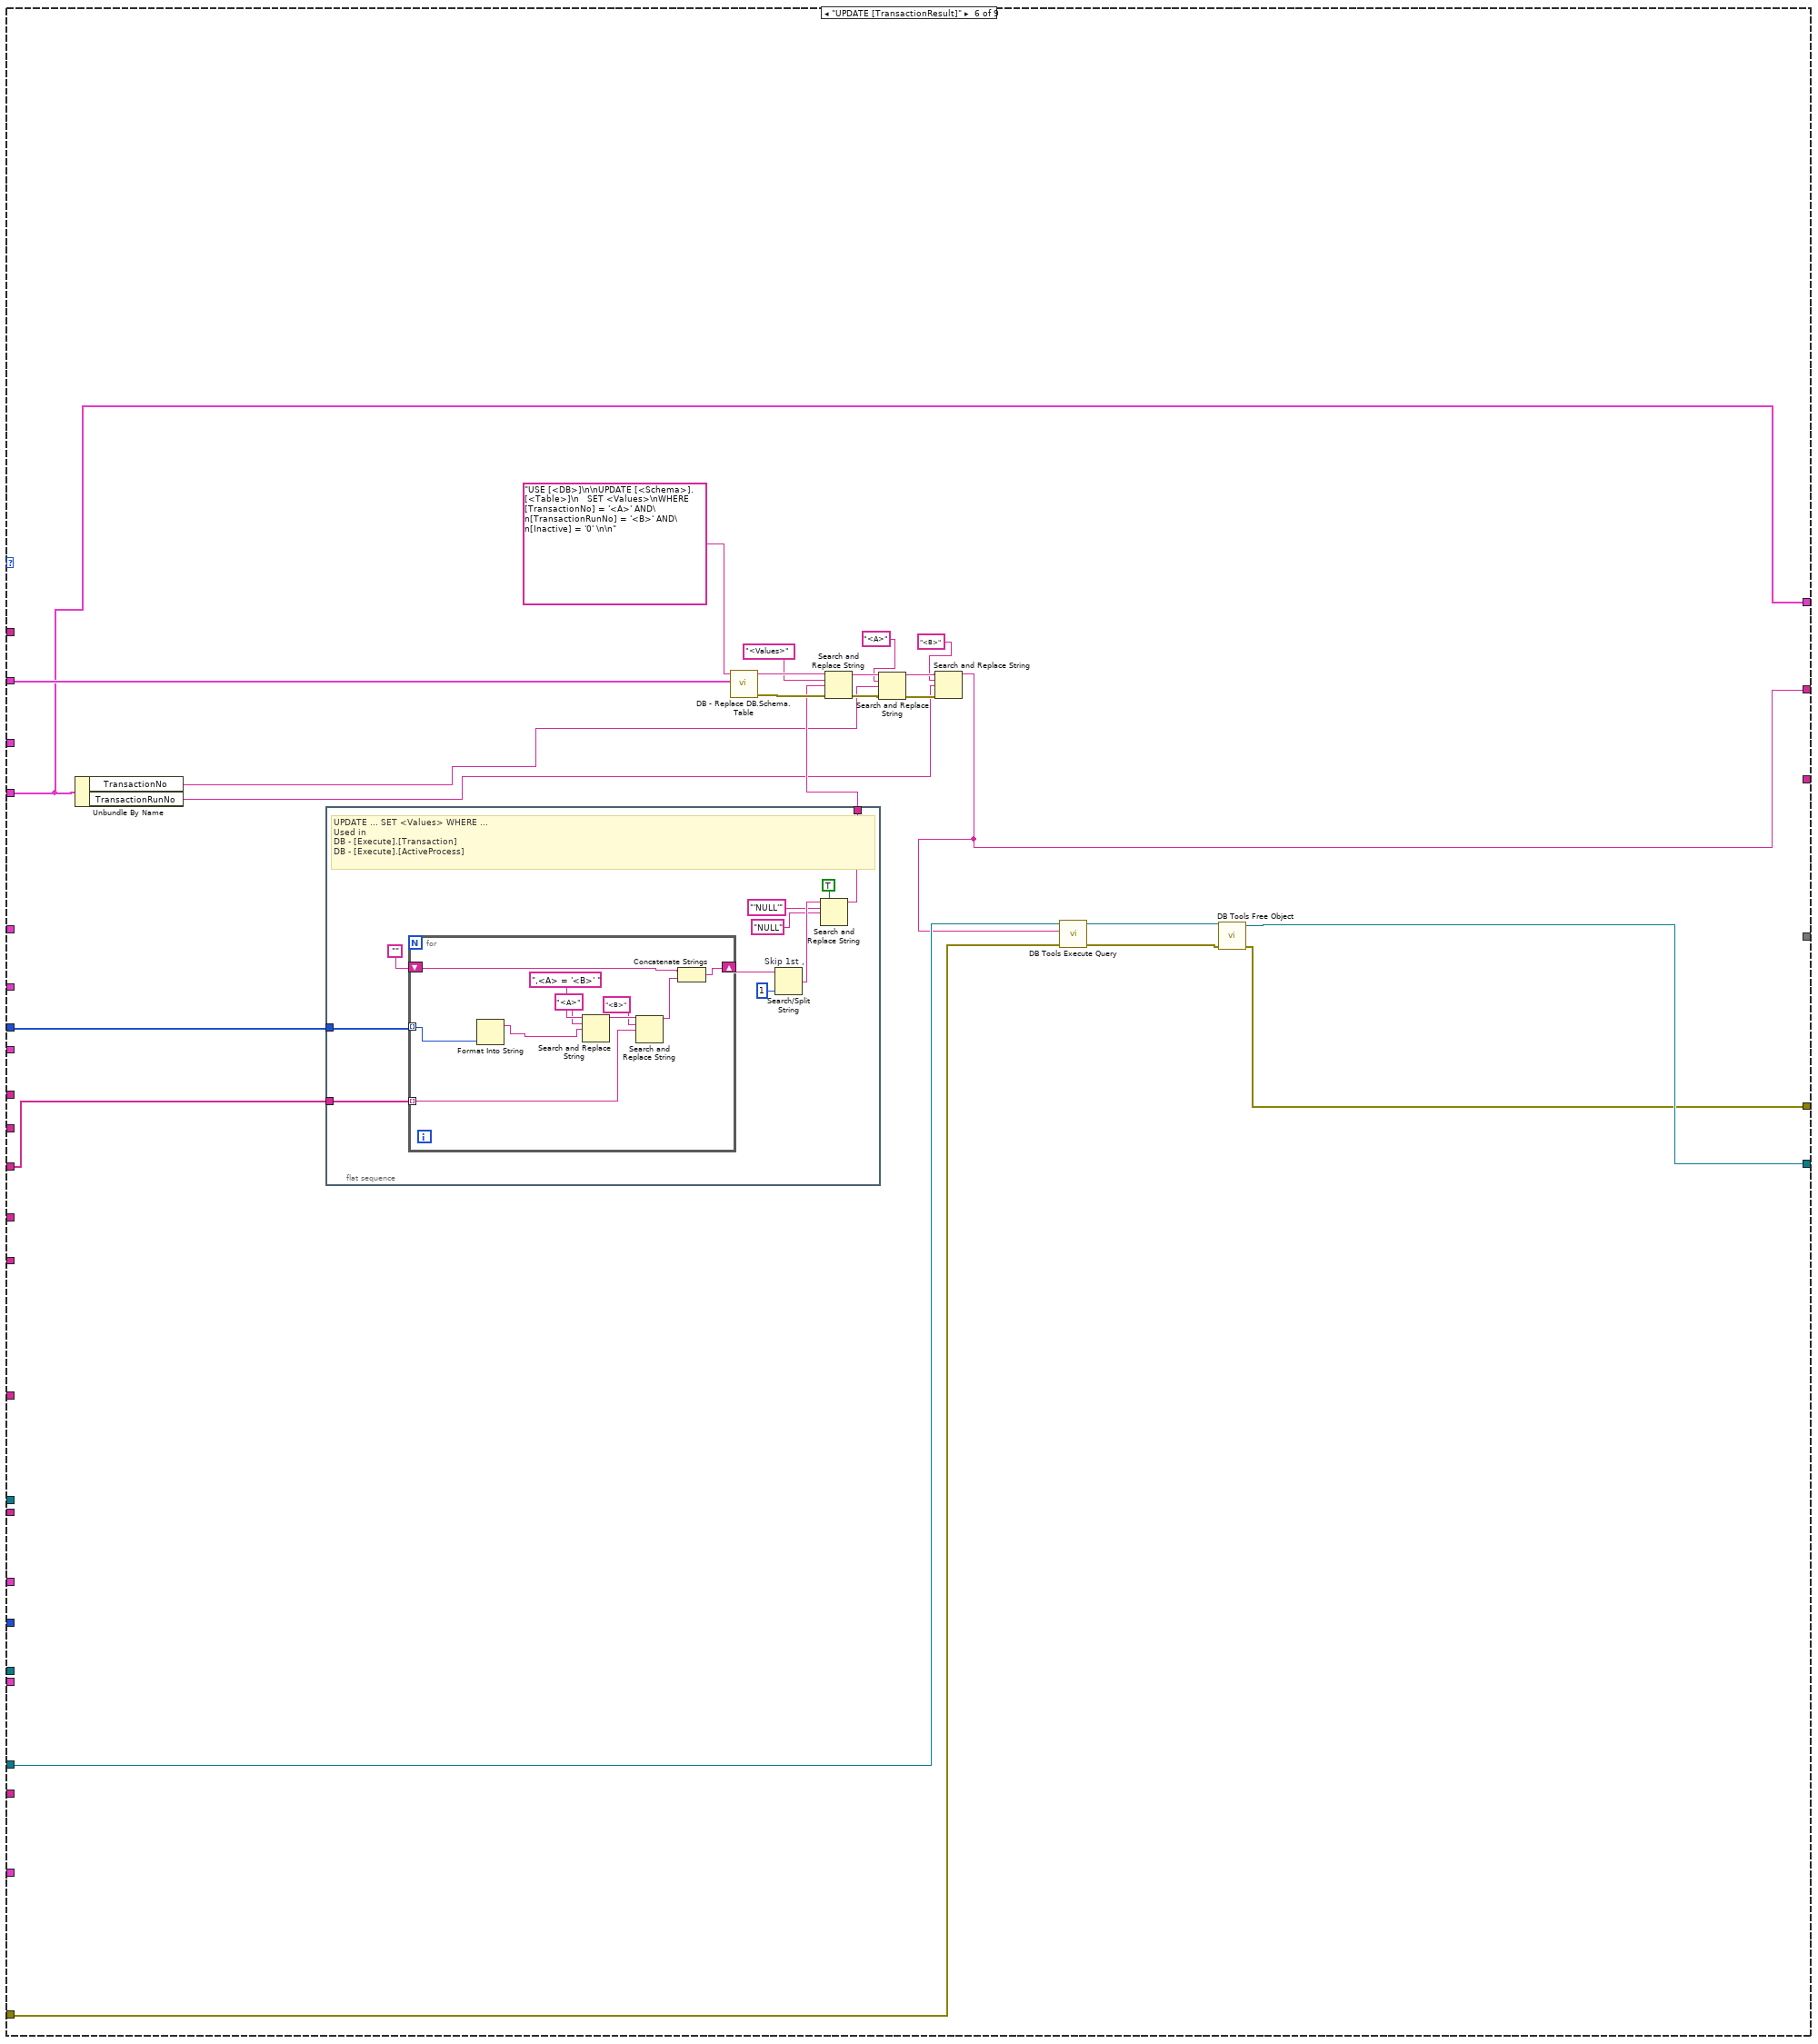
[diagram p7: hidden frame]
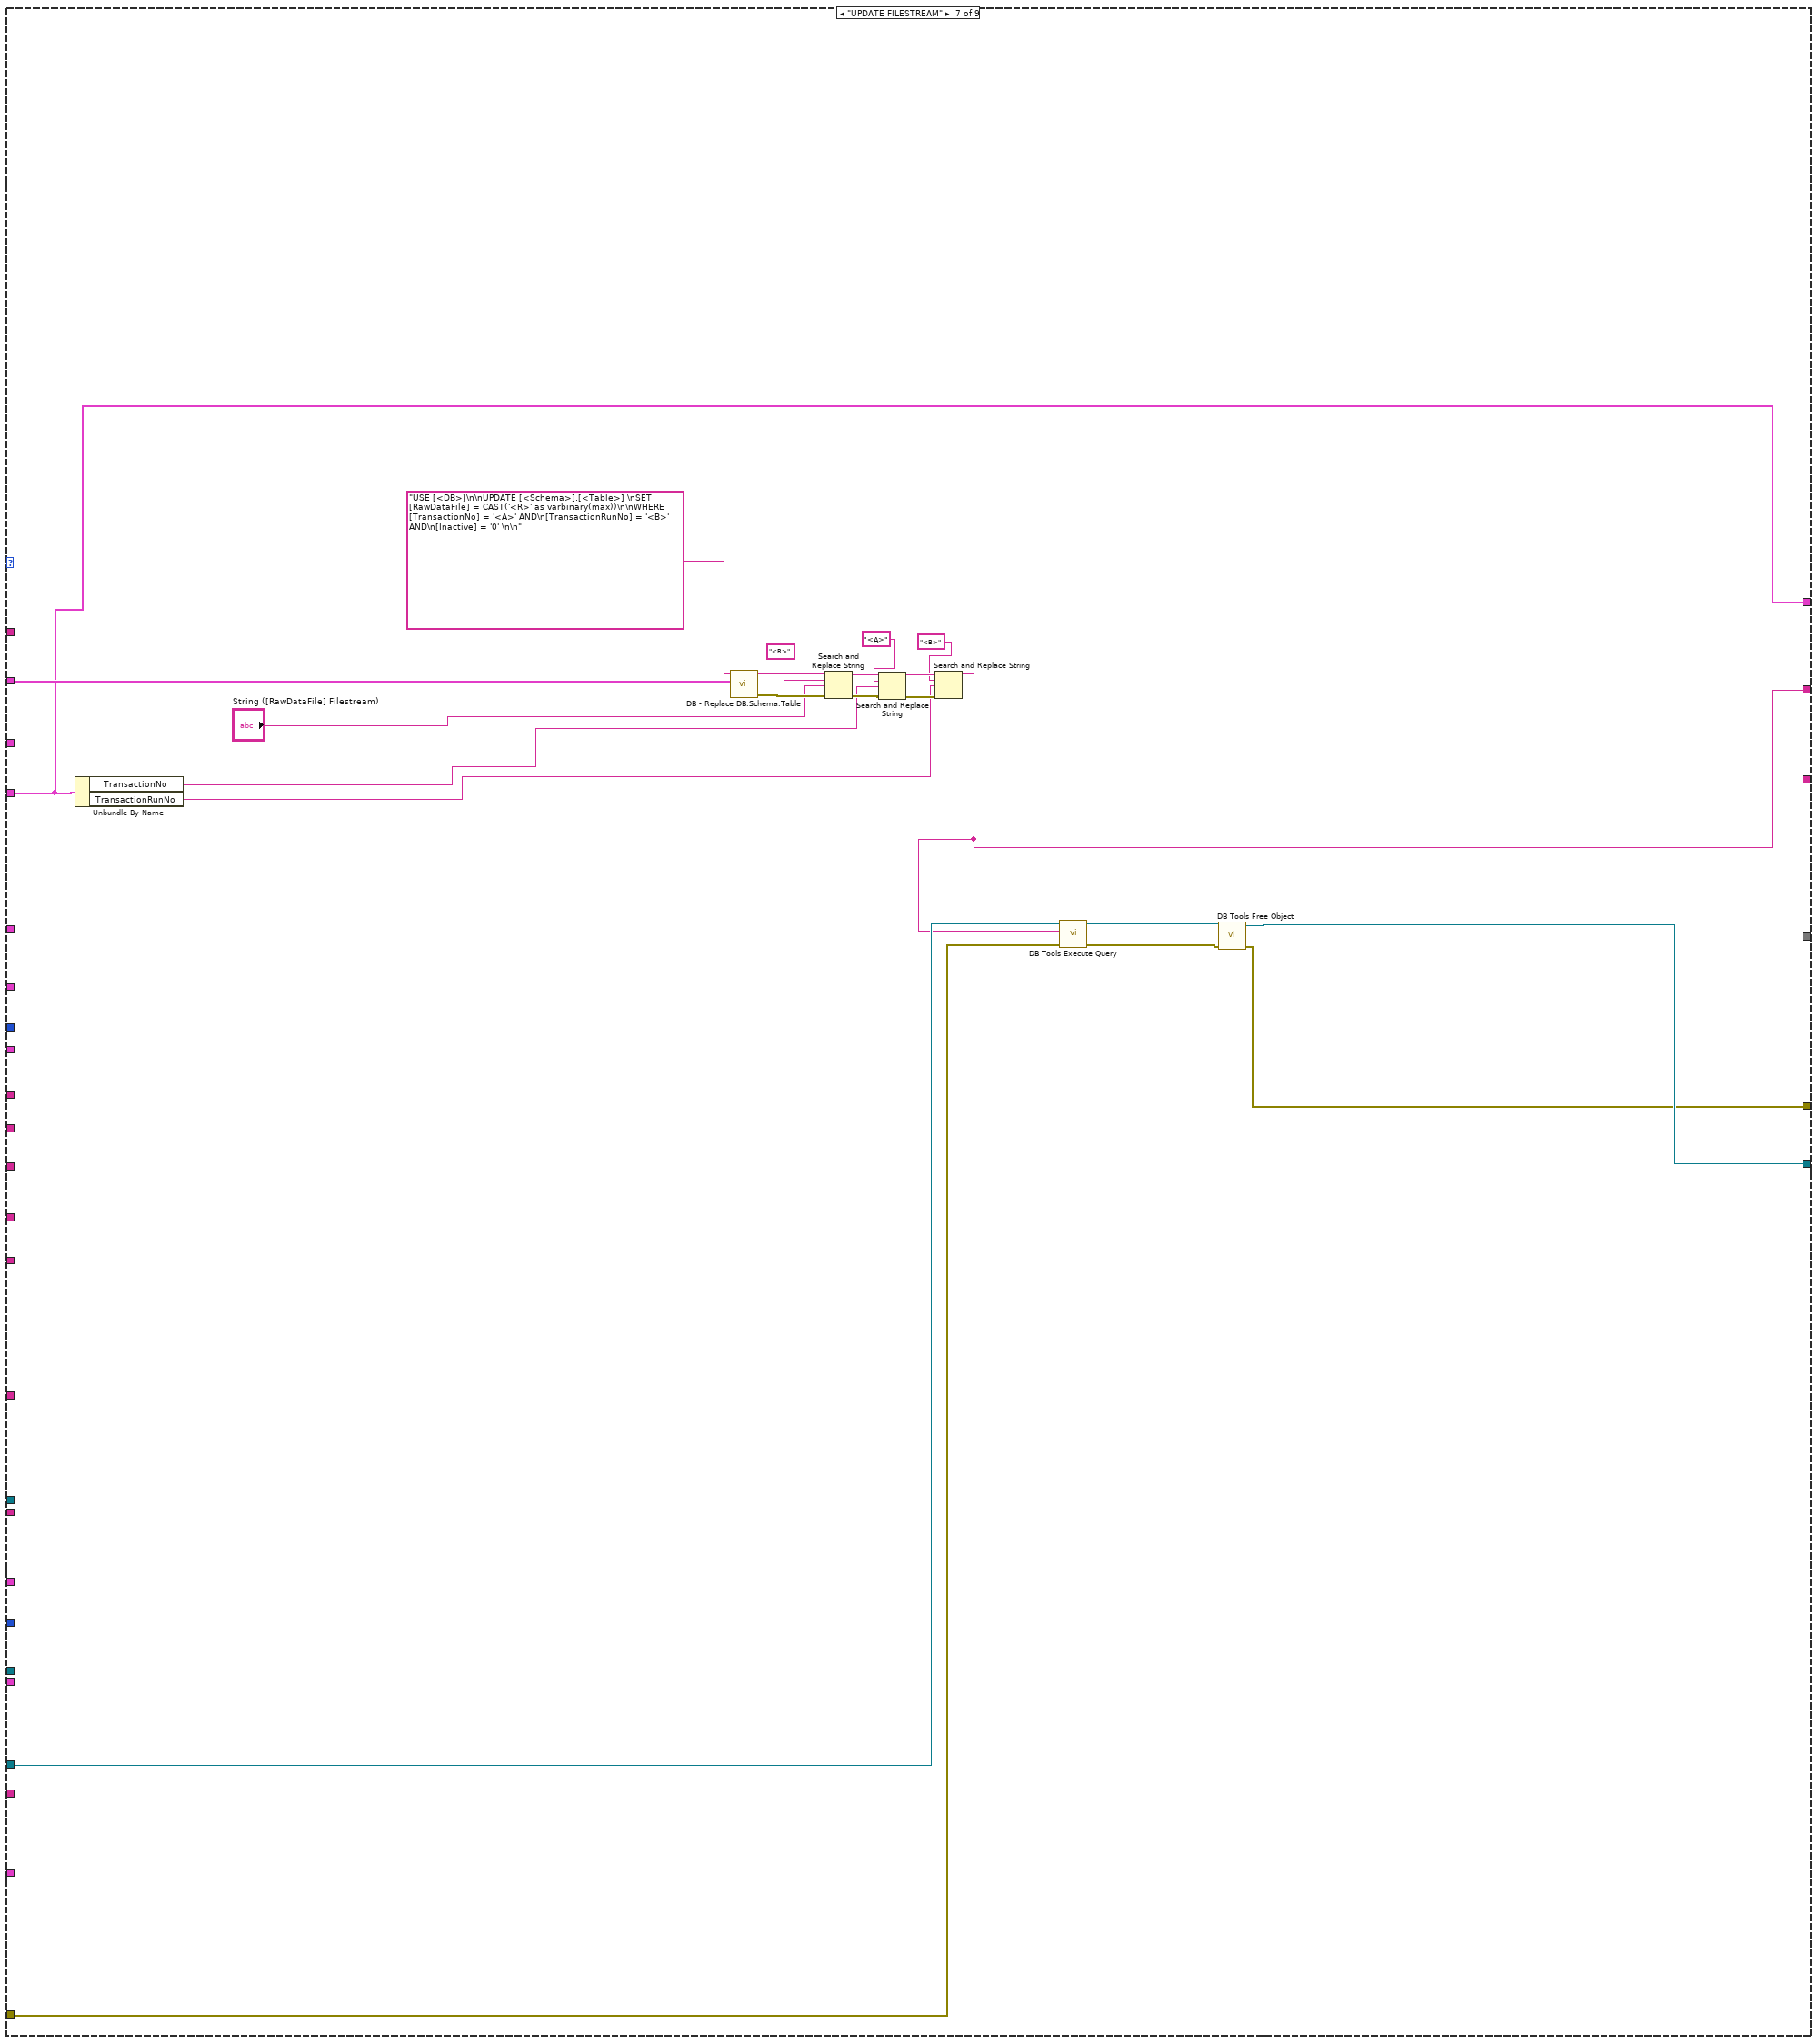
[diagram p8: hidden frame]
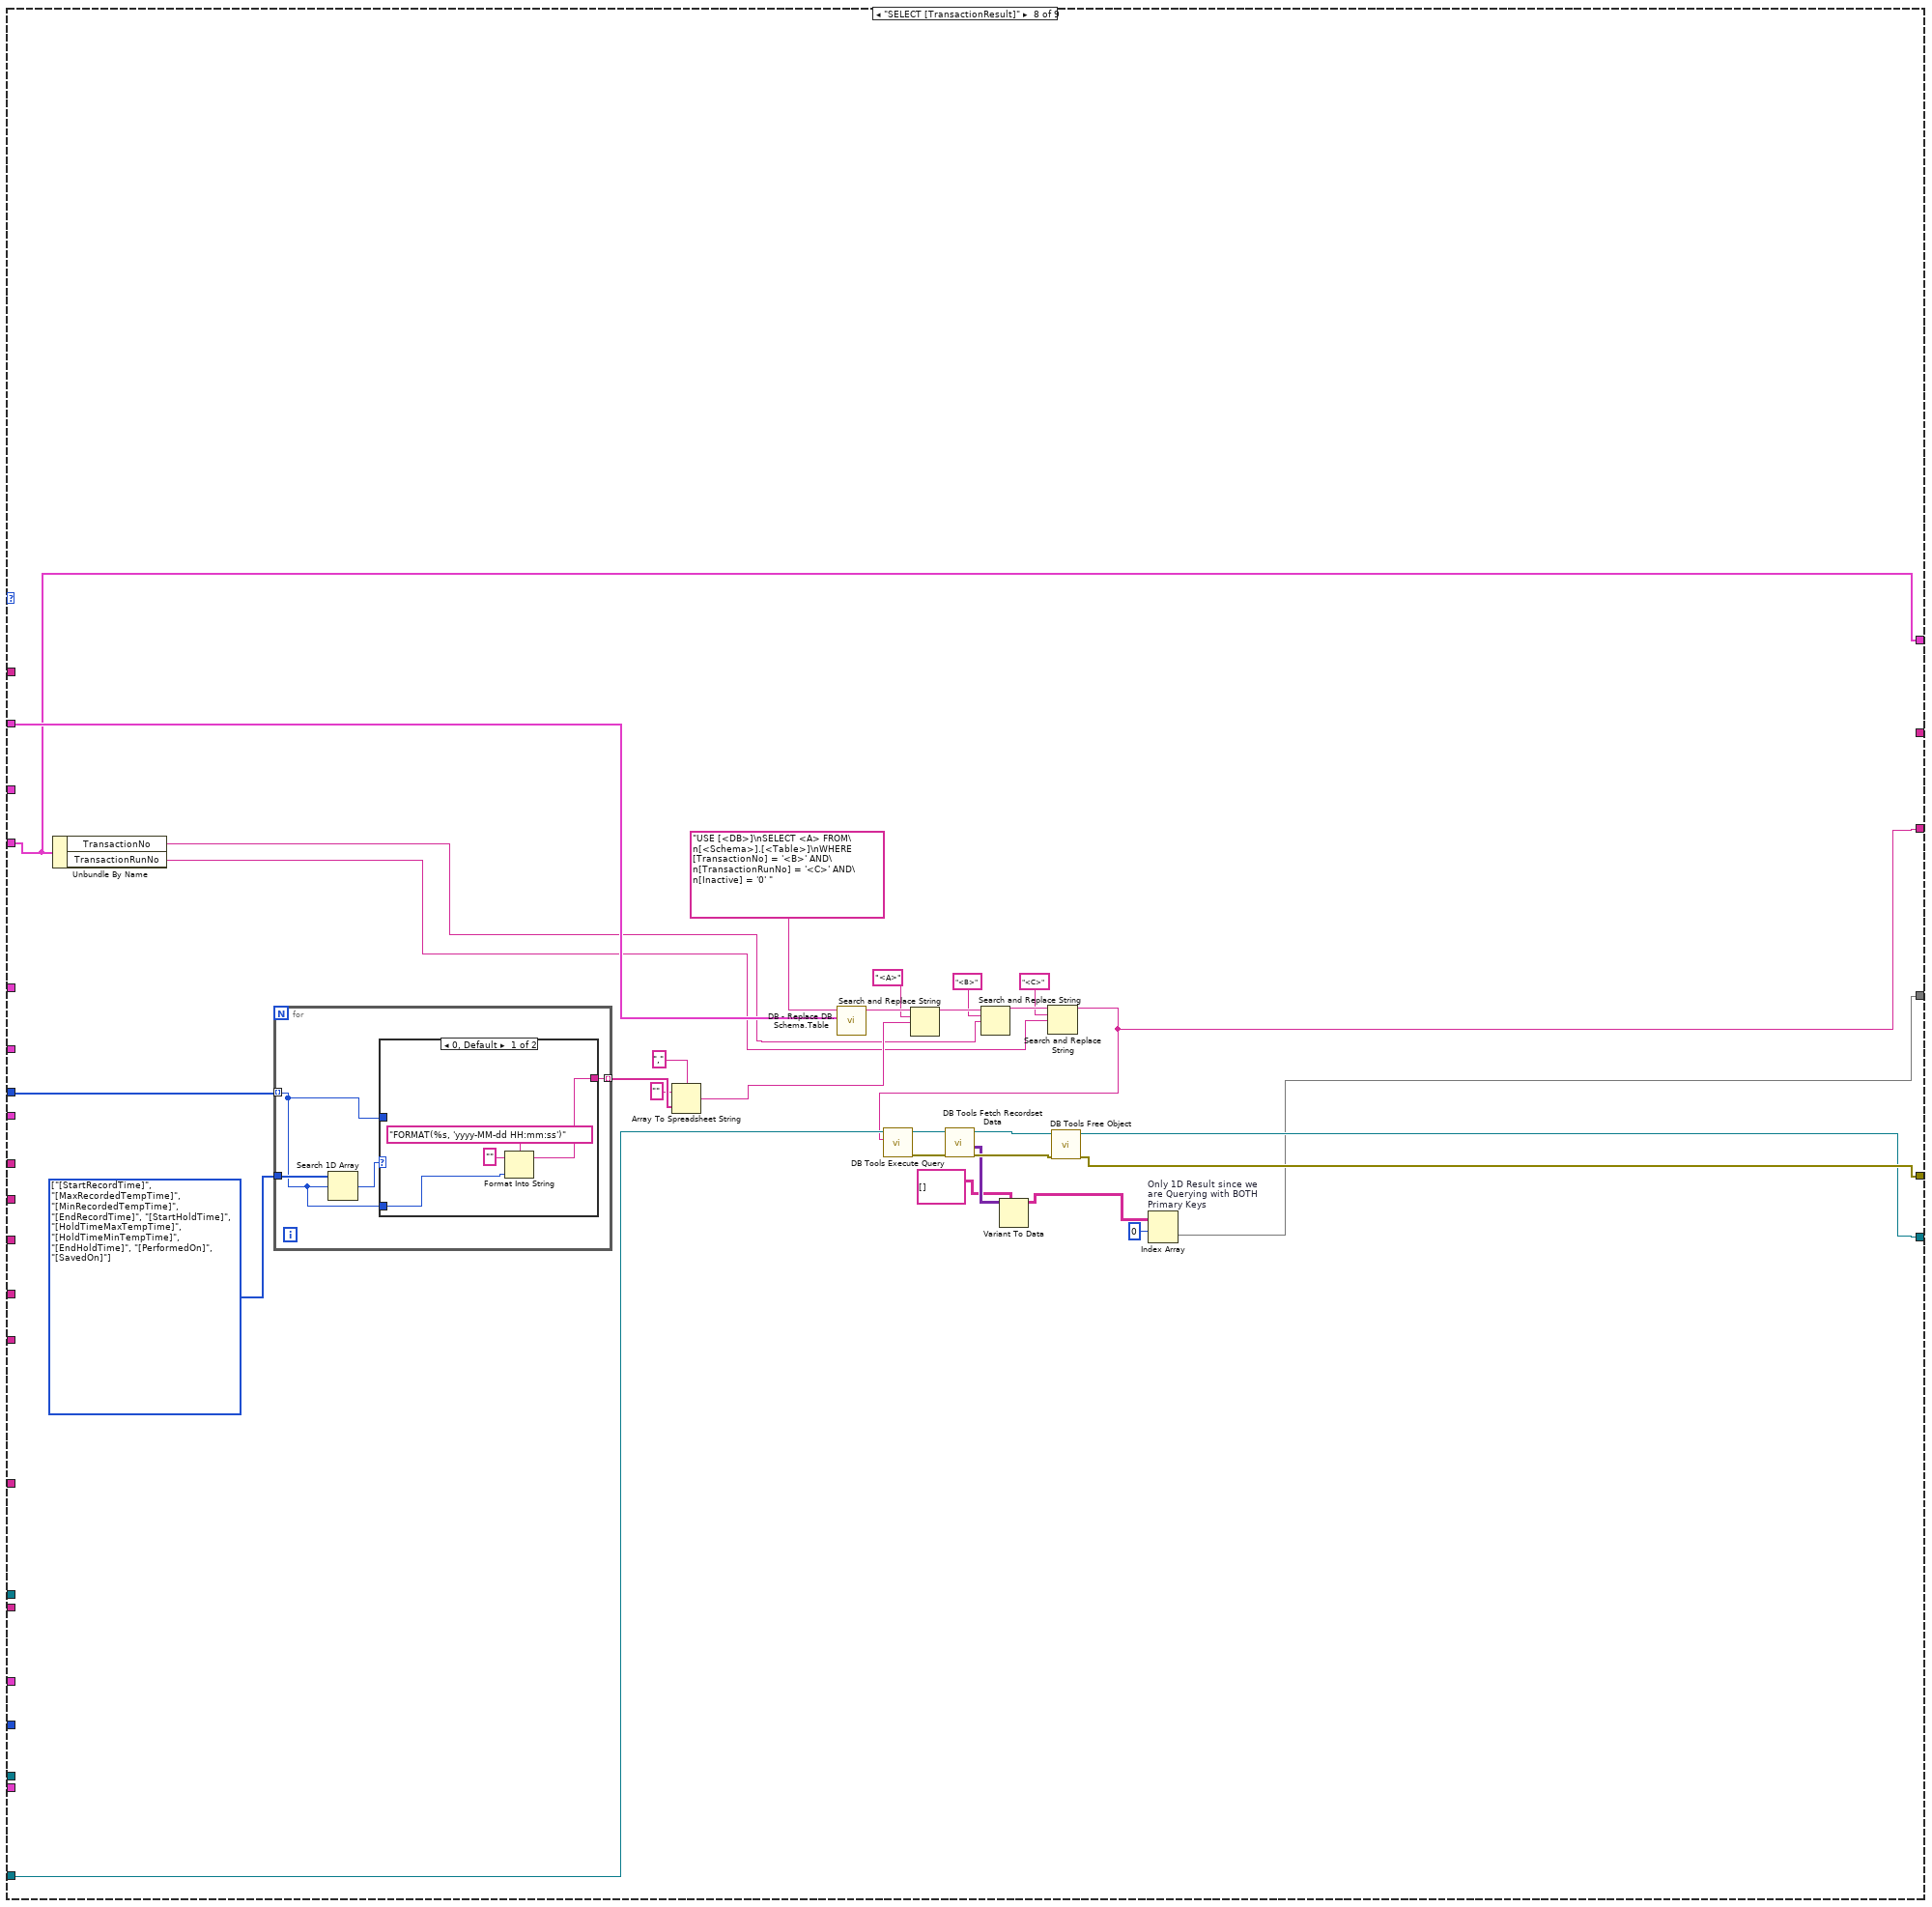
[diagram p9: hidden frame]
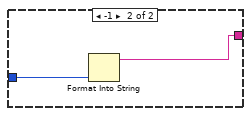
[diagram p10: hidden frame]
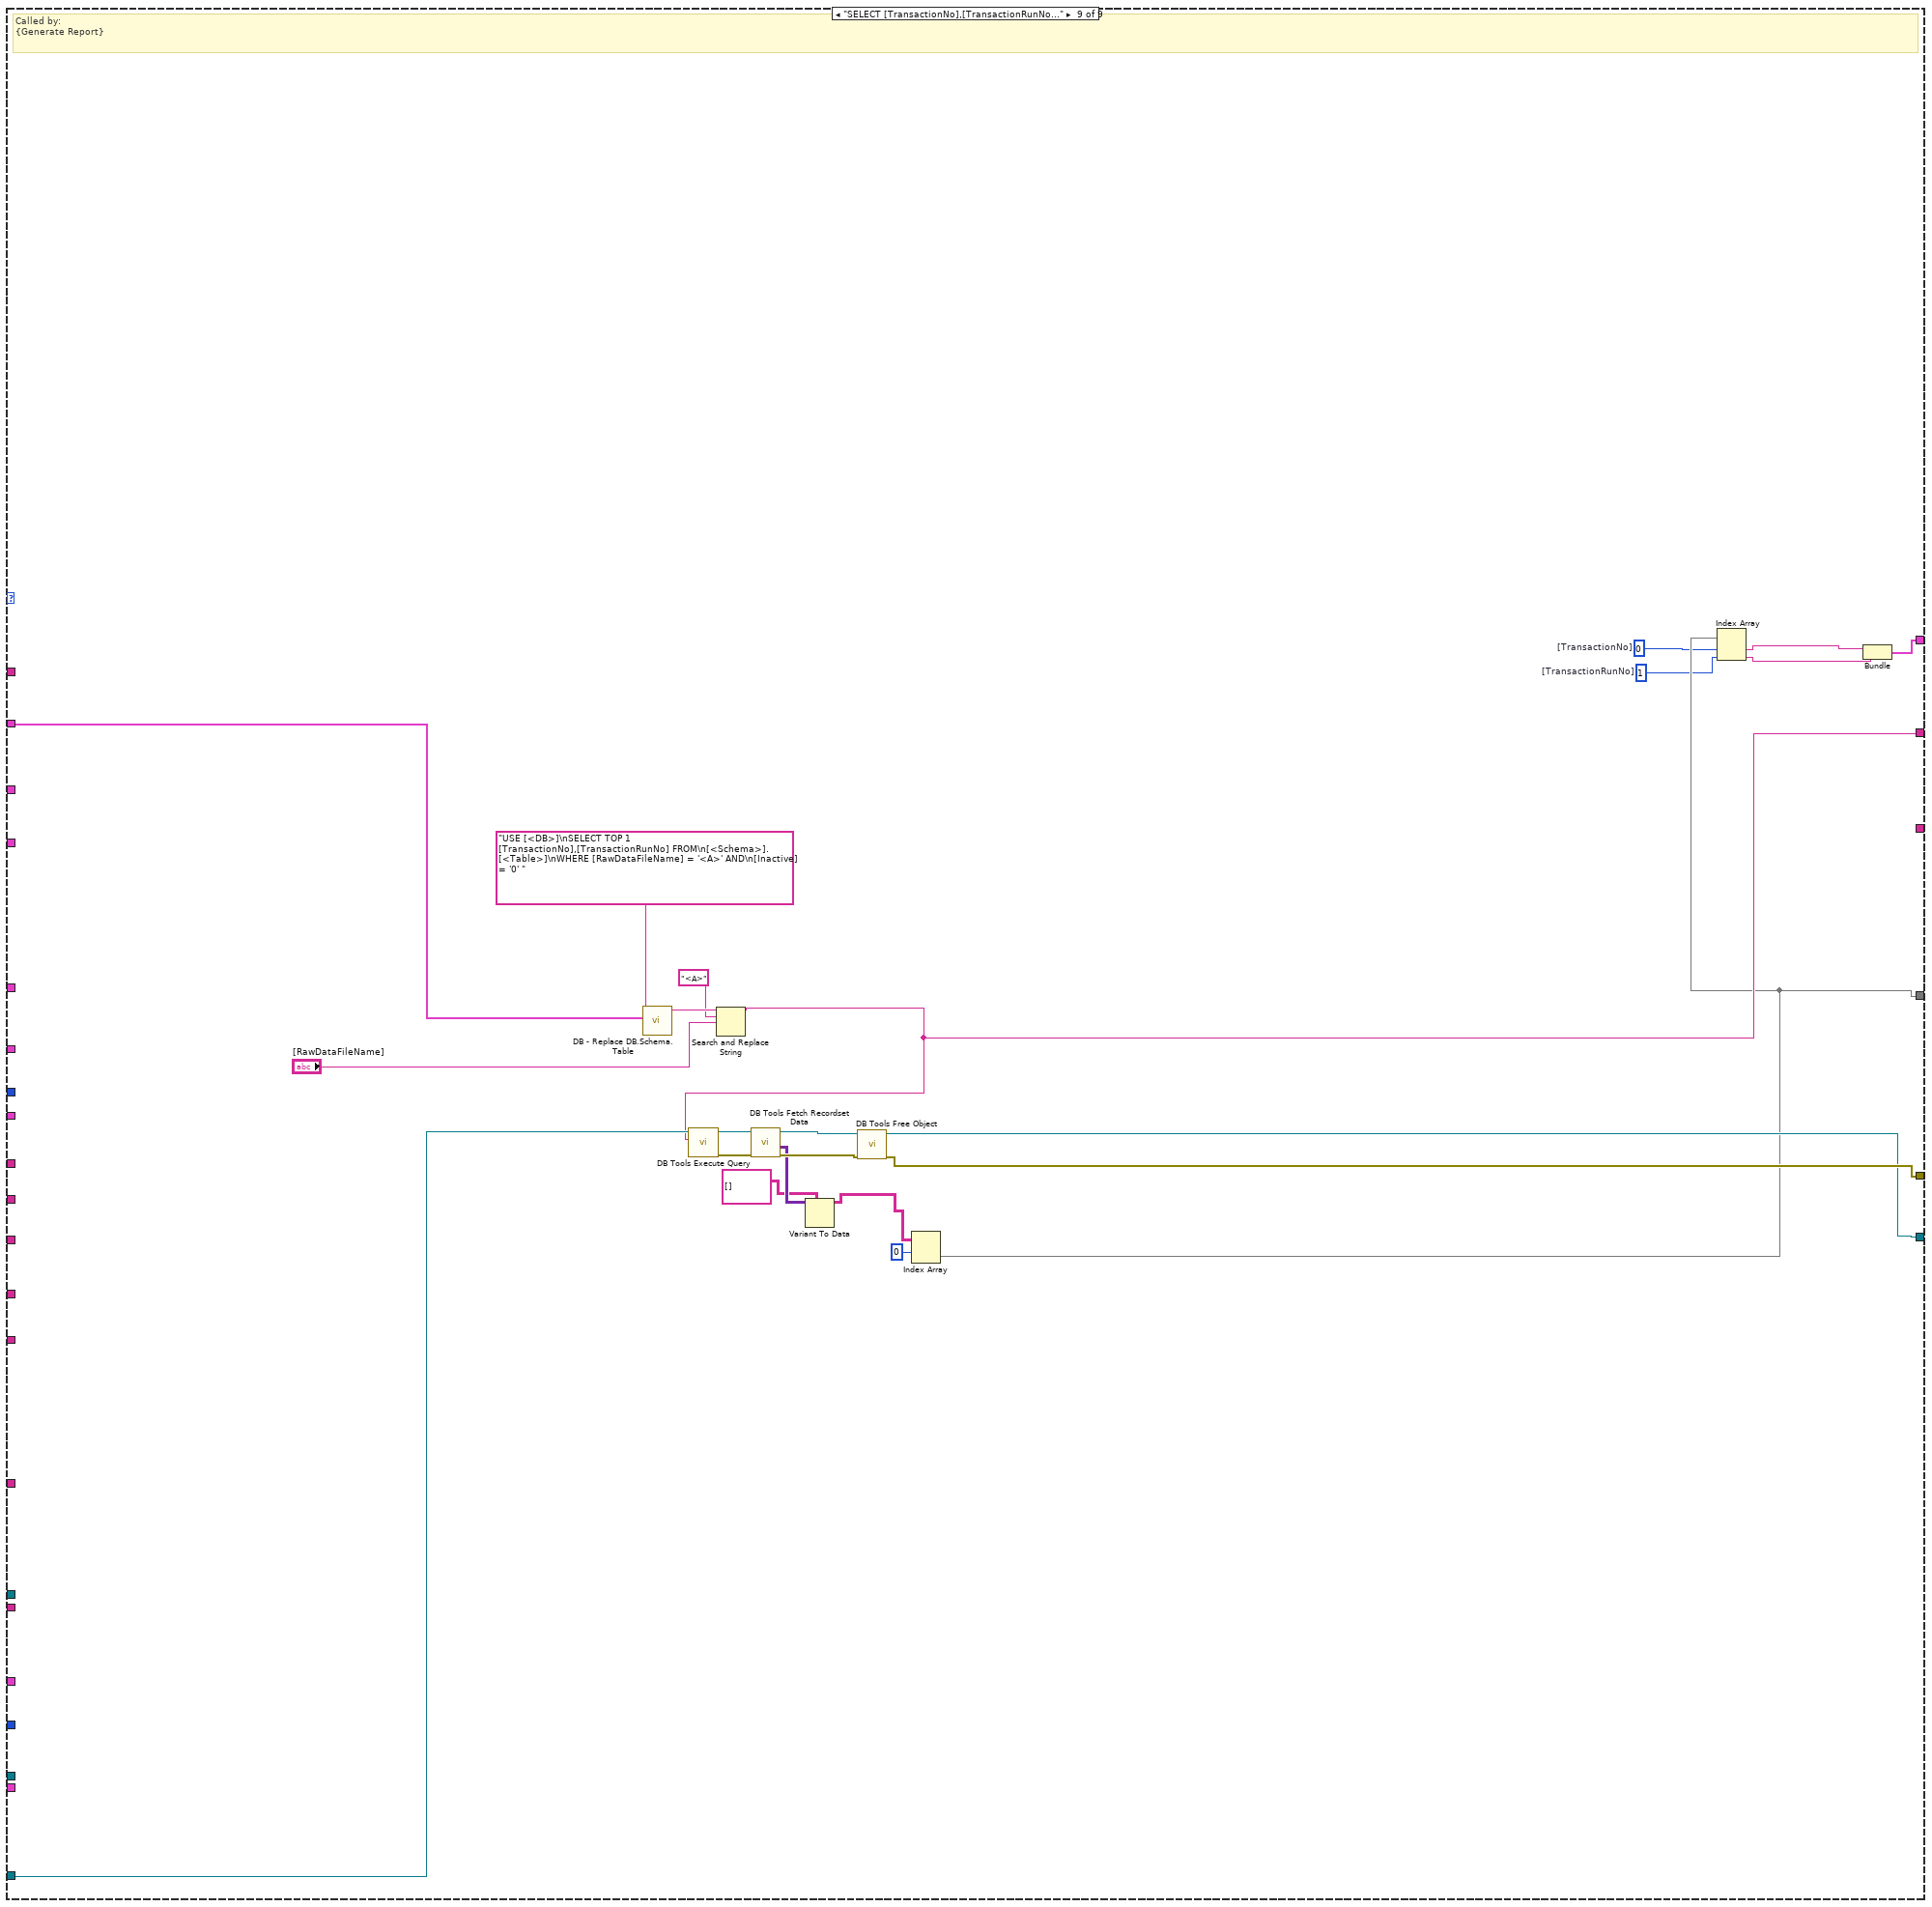
[diagram p11: hidden frame]
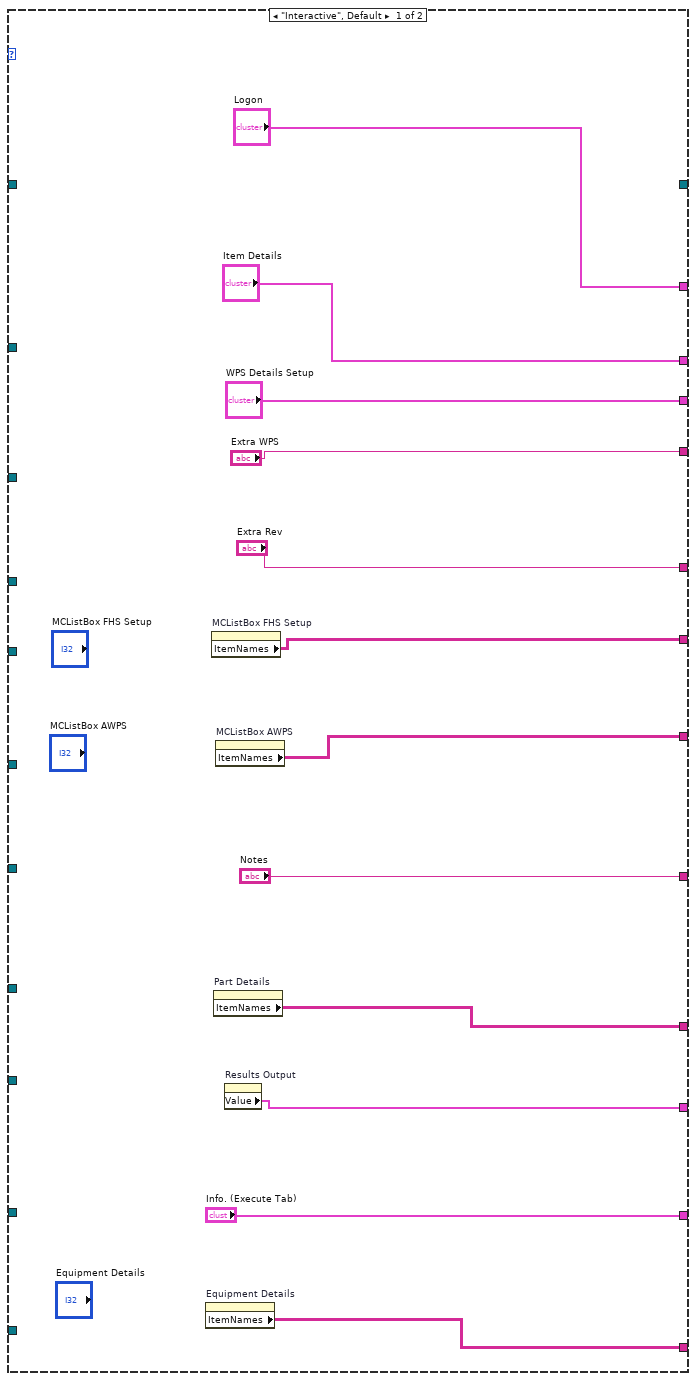
[diagram p12: hidden frame]
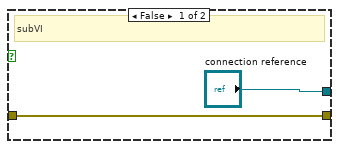
[diagram p14: hidden frame]
diagram:
  n1 = Unbundle By Name("Refnums") -> ("Item Details"=w28:refnum<vi>, "WPS Details"=w27:refnum<vi>, "WPS (Extra)"=w26:refnum<vi>, "Rev (Extra)"=w25:refnum<vi>, "FHS MCListbox"=w17:refnum<vi>, "Additional WPS/Ref MCListBox"=w24:refnum<vi>, "Notes"=w23:refnum<vi>, "Part Details (MClistBox)"=w22:refnum<vi>, "Result Output"=w7:refnum<vi>)
  n2 = Unbundle By Name("DB Refnums II") -> ("Info. (Execute Tab)"=w4:refnum<vi>, "CompactRIO Module Details"=w2:refnum<vi>)
  n3 = call "VI - Interactive or SubVI.vi"() -> ("Mode"=w31:T14)  [unwired: 5 in]
  n4 = call "VI - Interactive or SubVI.vi"() -> ("Mode"=w21:T14)  [unwired: 5 in]
  n5 = case shown="\"subVI Mode\"" w31 {
    tunnel: ["Item Details" w106] -> w36
    tunnel: ["Logon" w73] -> w38
    tunnel: ["WPS Details Setup" w105] -> w37
    tunnel: ["Extra Rev" w74] -> w35
    tunnel: ["Extra WPS" w75] -> w34
    tunnel: w24 -> [_ w82]
    tunnel: [w59 w104] -> w33
    tunnel: ["Notes" w96] -> w32
    tunnel: w28 -> [_ w86]
    tunnel: w26 -> [_ w84]
    tunnel: w23 -> [_ w81]
    tunnel: [_ w86] -> w30
    tunnel: w22 -> [_ w80]
    tunnel: [w55 w103] -> w29
    tunnel: w27 -> [_ w85]
    tunnel: w25 -> [_ w83]
    tunnel: w17 -> [_ w79]
    tunnel: [w54 w76] -> w18
    tunnel: w7 -> [_ w71]
    tunnel: [w53 w69] -> w6
    tunnel: w4 -> [_ w68]
    tunnel: ["Info. (Execute Tab)" w67] -> w3
    tunnel: w2 -> [_ w65]
    tunnel: [w51 w63] -> w1
    frame "Interactive", Default {
      n6 = property on="Equipment Details" class="MCListbox (strict)"() -> ("ItemNames"=w51:string[][])  [unwired: 2 in, 2 out]
      n7 = property on="MCListBox FHS Setup" class="MCListbox (strict)"() -> ("ItemNames"=w54:string[][])  [unwired: 2 in, 2 out]
      n8 = property on="Part Details" class="MCListbox (strict)"() -> ("ItemNames"=w55:string[][])  [unwired: 2 in, 2 out]
      n9 = property on="MCListBox AWPS" class="MCListbox (strict)"() -> ("ItemNames"=w59:string[][])  [unwired: 2 in, 2 out]
      n10 = property on="Results Output" class="Clust (strict)"() -> ("Value"=w53:cluster{"Output Set":T3, "Description":string})  [unwired: 2 in, 2 out]
    }
    frame "subVI Mode" {
      n11 = property class="MCListbox (strict)"(reference=w80) -> (error out=w87:errorcluster, "ItemNames"=w103:string[][])  [unwired: 1 in, 1 out]
      n12 = property class="MCListbox (strict)"(reference=w82) -> (error out=w98:errorcluster, "ItemNames"=w104:string[][])  [unwired: 1 in, 1 out]
      n13 = property class="MCListbox (strict)"(reference=w79) -> (error out=w78:errorcluster, "ItemNames"=w76:string[][])  [unwired: 1 in, 1 out]
      n14 = property class="Clust (strict)"(reference=w71) -> (error out=w72:errorcluster, "Value"=w69:cluster{"Output Set":T3, "Description":string})  [unwired: 1 in, 1 out]
      n15 = property class="Clust (strict)"(reference=w85) -> (error out=w101:errorcluster, "Value"=w105:T10)  [unwired: 1 in, 1 out]
      n16 = property class="Clust (strict)"(reference=w68) -> (error out=w66:errorcluster, "Value"=w67:T1)  [unwired: 1 in, 1 out]
      n17 = property class="MCListbox"(reference=w65) -> (error out=w64:errorcluster, "ItemNames"=w63:string[][])  [unwired: 1 in, 1 out]
      n18 = property class="Str"(reference=w81) -> (error out=w97:errorcluster, "Value"=w96:string)  [unwired: 1 in, 1 out]
      n19 = property class="Clust (strict)"(reference=w86) -> (error out=w102:errorcluster, "Value"=w106:T11)  [unwired: 1 in, 1 out]
      n20 = property class="Str"(reference=w84) -> (error out=w100:errorcluster, "Value"=w75:string)  [unwired: 1 in, 1 out]
      n21 = property class="Str"(reference=w83) -> (error out=w99:errorcluster, "Value"=w74:string)  [unwired: 1 in, 1 out]
      n22 = property on="Results Output" class="Clust (strict)"(error in=w72, "Value"=w69) -> (error out=w70:errorcluster)  [unwired: 1 in, 1 out]
      n23 = global read "Global SRTRS.vi" "Logon"() -> (w73:T9)
      n24 = property on="WPS Details Setup" class="Clust (strict)"(error in=w101, "Value"=w105) -> (error out=w94:errorcluster)  [unwired: 1 in, 1 out]
      n25 = property on="Extra Rev" class="Str"(error in=w99, "Value"=w74) -> (error out=w92:errorcluster)  [unwired: 1 in, 1 out]
      n26 = property on="Extra WPS" class="Str"(error in=w100, "Value"=w75) -> (error out=w93:errorcluster)  [unwired: 1 in, 1 out]
      n27 = property on="MCListBox AWPS" class="MCListbox (strict)"(error in=w98, "ItemNames"=w104) -> (error out=w91:errorcluster)  [unwired: 1 in, 1 out]
      n28 = property on="Notes" class="Str"(error in=w97, "Value"=w96) -> (error out=w90:errorcluster)  [unwired: 1 in, 1 out]
      n29 = property on="MCListBox FHS Setup" class="MCListbox (strict)"(error in=w78, "ItemNames"=w76) -> (error out=w77:errorcluster)  [unwired: 1 in, 1 out]
      n30 = property on="Part Details" class="MCListbox (strict)"(error in=w87, "ItemNames"=w103) -> (error out=w89:errorcluster)  [unwired: 1 in, 1 out]
      n31 = property on="Item Details" class="Clust (strict)"(error in=w102, "Value"=w106) -> (error out=w95:errorcluster)  [unwired: 1 in, 1 out]
      n32 = Merge Errors(w95, w94, w93, w92, w77, w91, w90, w89, w70, w66, w64) -> (→"Refnums error out":errorcluster)
    }
  }
  n33 = case shown="\"subVI Mode\"" w21 {
    tunnel: [w107 "error in (no error)"] -> w20
    frame "Interactive", Default {
      w107 = errorcluster {"status"=FALSE, "code"=0, "source"=""} ("error in (no error)")
      n34 = local write "error in (no error)"(w107) -> ()
    }
    frame "subVI Mode" {
    }
  }
  n35 = Unbundle By Name("DB Connection") -> ("Open"=w40:bool, "Close"=w39:bool)
  n36 = case shown="True" w40 {
    tunnel: ["connection reference" w114] -> w49
    tunnel: w20 -> [w109 w113]
    tunnel: [w109 w112] -> w47
    frame False {
      # "subVI"
    }
    frame True {
      n37 = global read "Global SRTRS.vi" "SRTRS Connection Information"() -> (w111:T15)
      "Connection Information" <- w111
      n38 = Unbundle By Name(w111) -> ("Connection"=w116:string, "Username"=w117:string, "Password"=w115:string)
      n39 = call-poly <vilib>:"DB Tools Open Connection.vi"("password"=w115, "userID"=w117, "error in (no error)"=w113, "connection information"=w116) -> ("error out"=w112:errorcluster, "connection reference"=w114:T12)  [unwired: 4 in]
    }
  }
  n40 = call "DB - Split DB.Schema.Table.vi"("DB.Schema.Table"="DB.Schema.Table 2\n(NA)") -> ("DB.Schema.Table"=w44:T16)  [unwired: 10 in]
  n41 = call "DB - Split DB.Schema.Table.vi"("DB.Schema.Table"="DB.Schema.Table") -> ("DB.Schema.Table"=w48:T16)  [unwired: 10 in]
  n42 = case shown="\"INSERT INTO [Header]\"" "DB - Execute Transaction" {
    tunnel: w49 -> [w184 w217 w243 w270 w317 w353 w396 w421 w459]
    tunnel: [w152 w215 w241 w268 w315 w351 w394 w413 w451] -> w42
    tunnel: [w155 w214 w240 w267 w314 w350 w393 w414 w452] -> w10
    tunnel: w48 -> [w175 w219 w247 w274 w318 w357 w400 w428 w462]
    tunnel: w47 -> [w151 w216 w242 w269 w316 w352 w395 _ _]
    tunnel: w30 -> [_ _ _ _ _ _ _ _ _]
    tunnel: w44 -> [_ _ _ _ _ _ _ _ _]
    tunnel: string[] ["OperationNo", "Qty", "NCRNo", "CustomerID", "Customer", "Project", "SalesOrderNo", "SalesOrderItemNo", "MaterialNo", "MaterialRev", "MaterialDesc", "SerialNos", "UnitOfQty"] -> [_ _ _ _ _ _ _ _ _]
    tunnel: w38 -> [w192 _ _ _ _ _ _ _ _]
    tunnel: w37 -> [w191 _ _ _ w291 _ _ _ _]
    tunnel: w36 -> [_ _ _ _ _ _ _ _ _]
    tunnel: w35 -> [w163 _ _ _ _ _ _ _ _]
    tunnel: w34 -> [w164 _ _ _ _ _ _ _ _]
    tunnel: w33 -> [w190 _ _ _ _ _ _ _ _]
    tunnel: w32 -> [w187 _ _ _ _ _ _ _ _]
    tunnel: w31 -> [_ _ _ _ _ _ _ _ _]
    tunnel: w29 -> [_ _ _ _ _ _ _ _ _]
    tunnel: "Refnums" -> [_ _ _ _ _ _ _ _ _]
    tunnel: w18 -> [_ _ _ _ w292 _ _ _ _]
    tunnel: w17 -> [_ _ _ _ _ _ _ _ _]
    tunnel: [w154 w209 w229 w258 w279 w341 w384 _ w449] -> w15
    tunnel: [w143 _ _ _ _ _ _ w412 _] -> w14
    tunnel: "[TransactionResult] v02" -> [_ _ _ _ _ w339 _ w430 _]
    tunnel: [w141 w208 w237 w266 w276 w336 w381 w405 w443] -> w12
    tunnel: "Transaction" -> [w140 w208 w237 w266 w276 w336 w381 w405 _]
    tunnel: "<Values>" -> [_ _ w225 w261 _ w335 _ _ _]
    tunnel: [_ _ _ w249 _ _ _ w402 w446] -> w8
    tunnel: w6 -> [w134 _ _ _ _ _ _ _ _]
    tunnel: w3 -> [w132 _ _ _ _ _ _ _ _]
    tunnel: w1 -> [w127 _ _ _ _ _ _ _ _]
    frame "INSERT INTO [Header]" {
      w126 = 5  # EquipmentID
      w118 = T17[] [enum."[Equipment1Id]", enum."[Equipment2Id]", enum."[Equipment3Id]", enum."[Equipment4Id]", enum."[Equipment5Id]", enum."[Equipment6Id]", enum."[Equipment7Id]", enum."[Equipment8Id]", enum."[Equipment9Id]", enum."[Equipment10Id]"] items=["[SystemId]", "[PlantId]", "[StationId]", "[ProcedureNo]", "[ProcedureRev]", "[WpsNo]", "[WpsRev]", "[HoldTemperature]", "[UnitOfTemperature]", "[HoldTime]", "[OutputSetId]", "[AdditionalProcs]", "[Equipment1Id]", "[Equipment2Id]", "[Equipment3Id]", "[Equipment4Id]", "[Equipment5Id]", "[Equipment6Id]", "[Equipment7Id]", "[Equipment8Id]", "[Equipment9Id]", "[Equipment10Id]", "[PermittedTempDiff]", "[PermittedTimeDiff]", "[Notes]", "[LastSavedBy]", "[LastSavedOn]", "[Indicator1]", "[Indicator2]", "[Remark1]", "[Remark2]", "[Remark3]", "[Remark4]", "[Inactive]"]
      w125 = T17[] [enum."[SystemId]", enum."[PlantId]", enum."[StationId]", enum."[ProcedureNo]", enum."[ProcedureRev]", enum."[WpsNo]", enum."[WpsRev]", enum."[HoldTemperature]", enum."[UnitOfTemperature]", enum."[HoldTime]", enum."[AdditionalProcs]", enum."[OutputSetId]", enum."[PermittedTempDiff]", enum."[PermittedTimeDiff]", enum."[Notes]", enum."[LastSavedBy]", enum."[LastSavedOn]"] items=["[SystemId]", "[PlantId]", "[StationId]", "[ProcedureNo]", "[ProcedureRev]", "[WpsNo]", "[WpsRev]", "[HoldTemperature]", "[UnitOfTemperature]", "[HoldTime]", "[OutputSetId]", "[AdditionalProcs]", "[Equipment1Id]", "[Equipment2Id]", "[Equipment3Id]", "[Equipment4Id]", "[Equipment5Id]", "[Equipment6Id]", "[Equipment7Id]", "[Equipment8Id]", "[Equipment9Id]", "[Equipment10Id]", "[PermittedTempDiff]", "[PermittedTimeDiff]", "[Notes]", "[LastSavedBy]", "[LastSavedOn]", "[Indicator1]", "[Indicator2]", "[Remark1]", "[Remark2]", "[Remark3]", "[Remark4]", "[Inactive]"]  # 2014-11-09 15:18
      w185 = "%Y-%m-%d %H:%M:%S"  # SQL Server datetime
      n43 = Unbundle By Name(w140) -> ("TransactionNo"=w139:string)
      n44 = Unbundle By Name(w132) -> ("Variant Allowed (Hold Temp)"=w131:dbl, "Variant Allowed (Hold Time)"=w130:dbl)
      n45 = Unbundle By Name(w192) -> ("PlantID"=w167:string, "SystemID"=w168:string, "UserID"=w186:string, "StationID"=w138:string)
      n46 = Unbundle By Name(w191) -> ("WPS/Ref"=w166:T3, "Rev"=w165:T3, "Hold Temperature"=w162:string, "WPS Details Temperature Units"=w161:string, "Hold Time (HH:MM)"=w160:string)
      n47 = call "DB - Replace DB.Schema.Table.vi"("error in (no error)"=w151, "DB.Schema.Table"=w175, "string in"="Use [<DB>]\n\nDECLARE @value as INT\nDECLARE @transactionNo as INT\nEXEC GetNewTransactionRunNo  @transactionNo = <A>\n, @transactionRunNo = @value OUTPUT") -> ("error out"=w194:errorcluster, "string out"=w195:string)  [unwired: 7 in]
      n48 = Unbundle By Name(w134) -> ("Output Set"=w133:T3)
      n49 = Array To Spreadsheet String(delimiter (Tab)=",", array=w190, 3:"" ("format string")) -> (spreadsheet string=w159:string)
      n50 = Index Array(array=w127, index (col)=w126) -> (element=w120:string[])  [unwired: 1 in]
      n51 = Search and Replace String(replace all?=TRUE ("replace all? (F)"), input string=w195, search string="<A>", replace string=w139, error in=w194) -> (result string=w154:string, error out=w150:errorcluster)  [unwired: 3 in, 2 out]
      n52 = call-poly <vilib>:"DB Tools Execute Query.vi"("error in (no error)"=w150, "SQL query"=w154, "connection reference"=w184) -> ("error out"=w177:errorcluster, "recordset reference"=w178:T18)  [unwired: 5 in]
      n53 = Number To Decimal String(number=w130) -> (decimal integer string=w128:string)  [unwired: 1 in]
      n54 = Number To Decimal String(number=w131) -> (decimal integer string=w129:string)  [unwired: 1 in]
      n55 = Format Date/Time String(time format string (%c)=w185) -> (date/time string=w183:string)  [unwired: 2 in]
      n56 = call-poly <vilib>:"DB Tools Fetch Element Data.vi"("error in (no error)"=w177, "column index"=0, "recordset reference"=w178) -> ("error out"=w180:errorcluster, "data"=w142:string, "recordset reference out"=w179:T18)  [unwired: 4 in]
      n57 = Bundle("TransactionNo"=w139, "data"=w142) -> (w141:cluster{"TransactionNo":string, "data":string})  [unwired: 1 in]
      n58 = call-poly <vilib>:"DB Tools Free Object.vi"("error in (no error)"=w180, "recordset reference"=w179) -> ("error out"=w156:errorcluster, "connection reference"=w153:T12)  [unwired: 8 in]
      n59 = Build Array(w129, w128, w187, w186, w183) -> (w157:string[])
      n60 = Build Array(w168, w167, w138, w166, w165, w164, w163, w162, w161, w160, w159, w133) -> (w158:T3[])
      n61 = Initialize Array("NULL", 10 ("dimension size")) -> (w121:string[])
      n62 = Replace Array Subset(array=w121, new element=w120) -> (w119:string[])  [unwired: 1 in]
      n63 = Build Array (concatenate)(w158, w157, w119) -> (w137:T3[])
      n64 = Build Array (concatenate)(w125, w118) -> (w124:T17[])
      n65 = call "DB - Replace DB.Schema.Table.vi"("error in (no error)"=w156, "DB.Schema.Table"=w175, "string in"="USE [<DB>]\n\nUPDATE [<Schema>].[<Table>]\n   SET <Values>\nWHERE [TransactionNo] = '<A>' AND\n[TransactionRunNo] = '<B>' \n\n") -> ("error out"=w173:errorcluster, "string out"=w174:string)  [unwired: 7 in]
      n66 = for {
        tunnel: w124 -> [w198] mode=indexing
        tunnel: [w197] -> w136 mode=indexing
        n67 = Format Into String(w198) -> (resulting string=w197:string)  [unwired: 3 in, 1 out]
      }
      n68 = Search and Replace String(input string=w174, search string="<A>", replace string=w139, error in=w173) -> (result string=w171:string, error out=w170:errorcluster)  [unwired: 4 in, 2 out]
      n69 = Search and Replace String(input string=w171, search string="<B>", replace string=w142, error in=w170) -> (result string=w147:string, error out=w145:errorcluster)  [unwired: 4 in, 2 out]
      n70 = call "DB - Update [Table] Set [ColNames] equ Data.vi"("<Data> (0xFFFE autodetect)"=w137, "[ColumnNames]"=w136) -> ("<Values>"=w135:string)  [unwired: 9 in]
      n71 = Search and Replace String(input string=w147, search string="<Values>", replace string=w135, error in=w145) -> (result string=w143:string, error out=w144:errorcluster)  [unwired: 4 in, 2 out]
      n72 = call-poly <vilib>:"DB Tools Execute Query.vi"("error in (no error)"=w144, "SQL query"=w143, "connection reference"=w153) -> ("error out"=w148:errorcluster, "recordset reference"=w149:T18)  [unwired: 5 in]
      n73 = call-poly <vilib>:"DB Tools Free Object.vi"("error in (no error)"=w148, "recordset reference"=w149) -> ("error out"=w155:errorcluster, "connection reference"=w152:T12)  [unwired: 8 in]
    }
    frame "INSERT INTO [TransactionResult]" {
      n74 = Unbundle By Name(w208) -> ("TransactionNo"=w200:string, "TransactionRunNo"=w199:string)
      n75 = Build Array(w200, w199) -> (w211:string[])
      n76 = call "DB - Array to Values.vi"("Array (0xFFFE autodetect)"=w211) -> ("<Values>"=w210:string)  [unwired: 10 in]
      n77 = call "DB - Replace DB.Schema.Table.vi"("DB.Schema.Table"=w219, "string in"="USE [<DB>]\n\nIF EXISTS(SELECT  1  FROM [<Schema>].[<Table>] \n     WHERE  [TransactionNo] = '<A>'  AND [TransactionRunNo] = '<B>')\n\nBEGIN\nDELETE FROM [<Schema>].[<Table>] \n      WHERE [TransactionNo] = '<A>'  AND [TransactionRunNo] = '<B>'\nEND\n\nINSERT INTO [<Schema>].[<Table>]\n           ([TransactionNo]\n           ,[TransactionRunNo]\n         ) \nVALUES (<Values>)\n\n") -> ("string out"=w207:string)  [unwired: 8 in, 1 out]
      n78 = Search and Replace String(replace all?=TRUE ("replace all? (F)"), input string=w207, search string="<A>", replace string=w200) -> (result string=w206:string)  [unwired: 4 in, 3 out]
      n79 = Search and Replace String(replace all?=TRUE ("replace all? (F)"), input string=w206, search string="<B>", replace string=w199) -> (result string=w205:string)  [unwired: 4 in, 3 out]
      n80 = Search and Replace String(input string=w205, search string="<Values>", replace string=w210) -> (result string=w209:string)  [unwired: 5 in, 3 out]
      n81 = call-poly <vilib>:"DB Tools Execute Query.vi"("error in (no error)"=w216, "SQL query"=w209, "connection reference"=w217) -> ("error out"=w212:errorcluster, "recordset reference"=w213:T18)  [unwired: 5 in]
      n82 = call-poly <vilib>:"DB Tools Free Object.vi"("error in (no error)"=w212, "recordset reference"=w213) -> ("error out"=w214:errorcluster, "connection reference"=w215:T12)  [unwired: 8 in]
    }
    frame "INSERT/UPDATE [Execute].[Active]" {
      n83 = Index Array(array=w225) -> (element #1=w224:string, element #2=w223:string, element #3=w222:string, element #4=w221:string)  [unwired: 4 in]
      n84 = call "DB - Replace DB.Schema.Table.vi"("DB.Schema.Table"=w247, "string in"="USE [<DB>]\nIF EXISTS\t(SELECT TOP 1 [TransactionNo],[TransactionRunNo] FROM [<Schema>].[<Table>] \n\t\t\t\tWHERE [PlantId] = '<A>' AND [StationId] = '<B>' AND [Inactive] = '0')\n\n\t\t\t\tBEGIN\n\t\t\t\tUPDATE [Execute].[Active] \n\t\t\t\tSET [TransactionNo] = '<C>',\n\t\t\t\t[TransactionRunNo] = '<D>'\n\t\t\t\tWHERE [PlantId] = '<A>' AND [StationId] = '<B>'\n\t\t\t\tEND\n\t\t\t\tELSE\n\t\t\t\tBEGIN\n\t\t\t\tINSERT INTO [<Schema>].[<Table>] \n\t\t\t\t([PlantId],[StationId],[TransactionNo],[TransactionRunNo])\n\t\t\t\tVALUES\n\t\t\t\t('<A>', '<B>', '<C>', '<D>')\n\t\t\t\tEND") -> ("error out"=w245:errorcluster, "string out"=w246:string)  [unwired: 8 in]
      n85 = Search and Replace String(replace all?=TRUE ("replace all? (F)"), input string=w246, search string="<A>", replace string=w224, error in=w245) -> (result string=w228:string)  [unwired: 3 in, 3 out]
      n86 = Search and Replace String(replace all?=TRUE ("replace all? (F)"), input string=w228, search string="<B>", replace string=w223) -> (result string=w227:string)  [unwired: 4 in, 3 out]
      n87 = Search and Replace String(replace all?=TRUE ("replace all? (F)"), input string=w227, search string="<C>", replace string=w222) -> (result string=w226:string)  [unwired: 4 in, 3 out]
      n88 = Search and Replace String(replace all?=TRUE ("replace all? (F)"), input string=w226, search string="<D>", replace string=w221) -> (result string=w229:string)  [unwired: 4 in, 3 out]
      n89 = call-poly <vilib>:"DB Tools Execute Query.vi"("error in (no error)"=w242, "SQL query"=w229, "connection reference"=w243) -> ("error out"=w238:errorcluster, "recordset reference"=w239:T18)  [unwired: 5 in]
      n90 = call-poly <vilib>:"DB Tools Free Object.vi"("error in (no error)"=w238, "recordset reference"=w239) -> ("error out"=w240:errorcluster, "connection reference"=w241:T12)  [unwired: 8 in]
    }
    frame "SELECT [Execute].[Active]" {
      n91 = Index Array(array=w261) -> (element #1=w260:string, element #2=w259:string)  [unwired: 4 in, 2 out]
      n92 = call "DB - Replace DB.Schema.Table.vi"("DB.Schema.Table"=w274, "string in"="USE [<DB>]\nSELECT [TransactionNo],[TransactionRunNo] FROM [<Schema>].[<Table>] \n\t\t\t\tWHERE [PlantId] = '<A>' AND [StationId] = '<B>' AND [Inactive] = '0'\n") -> ("error out"=w272:errorcluster, "string out"=w273:string)  [unwired: 8 in]
      n93 = Search and Replace String(replace all?=TRUE ("replace all? (F)"), input string=w273, search string="<A>", replace string=w260, error in=w272) -> (result string=w262:string)  [unwired: 3 in, 3 out]
      n94 = Search and Replace String(replace all?=TRUE ("replace all? (F)"), input string=w262, search string="<B>", replace string=w259) -> (result string=w258:string)  [unwired: 4 in, 3 out]
      n95 = call-poly <vilib>:"DB Tools Execute Query.vi"("error in (no error)"=w269, "SQL query"=w258, "connection reference"=w270) -> ("error out"=w252:errorcluster, "recordset reference"=w255:T18)  [unwired: 5 in]
      n96 = call-poly <vilib>:"DB Tools Fetch Recordset Data.vi"("error in (no error)"=w252, "recordset reference"=w255) -> ("error out"=w254:errorcluster, "recordset data"=w257:variant[][], "recordset reference out"=w253:T18)  [unwired: 3 in]
      n97 = Variant To Data(type=string[][] [], Variant=w257) -> (data=w251:string[][])  [unwired: 1 in, 1 out]
      n98 = call-poly <vilib>:"DB Tools Free Object.vi"("error in (no error)"=w254, "recordset reference"=w253) -> ("error out"=w267:errorcluster, "connection reference"=w268:T12)  [unwired: 8 in]
      n99 = Index Array(array=w251, index (row)=0) -> (element=w249:string[])  [unwired: 1 in]
    }
    frame "INSERT INTO [ProcedureItem]" {
      w303 = TRUE ("replace all? (F)")
      n100 = Unbundle By Name(w291) -> ("WPS Details Temperature Units"=w290:string)
      n101 = Unbundle By Name(w276) -> ("TransactionNo"=w278:string, "TransactionRunNo"=w277:string)
      n102 = Array Size(array=w292) -> (size(s)=w299:i32[])
      n103 = Index Array(array=w299) -> (element=w300:i32)  [unwired: 1 in]
      n104 = Decrement "Exclude Last Row (which is blank)"(x=w300) -> (x-1=w301:i32)
      n105 = for {
        N: w301 -> [_]
        tunnel: w292 -> [w326] mode=indexing
        shift-right: [w329] -> w294
        shift-left: "" -> [w330]
        tunnel: w290 -> [w325]
        w320 = "<D>"  # TransactionRunNo
        w321 = "<C>"  # TransactionNo
        w323 = "0"  # Inactive
        w327 = 2  # unitRampRate
        n106 = Insert Into Array(array=w326, index=w327, new element=w325) -> (w324:string[])
        n107 = Build Array (concatenate)(w321, w320, w324, w323) -> (w322:string[])
        n108 = Array To Spreadsheet String(delimiter (Tab)="','", array=w322, 3:"" ("format string")) -> (spreadsheet string=w328:string)
        n109 = Concatenate Strings(w330, ",('" ("string"), w328, "')" ("string")) -> (w329:string)
      }
      n110 = Build Array(w278, w277) -> (w311:string[])
      n111 = call "DB - Array to Values.vi"("Array (0xFFFE autodetect)"=w311) -> ()  [unwired: 10 in, 1 out]
      n112 = call "DB - Replace DB.Schema.Table.vi"("DB.Schema.Table"=w318, "string in"="USE [<DB>]\n\nIF EXISTS(SELECT 1 from [<Schema>].[<Table>] \n     WHERE  [TransactionNo] = '<A>'  AND [TransactionRunNo] = '<B>')\n\nBEGIN\nDELETE FROM [<Schema>].[<Table>] \n      WHERE [TransactionNo] = '<A>'  AND [TransactionRunNo] = '<B>'\nEND\n\nINSERT INTO [<Schema>].[<Table>]\n           ([TransactionNo]\n           ,[TransactionRunNo]\n           ,[SequenceNo]\n           ,[RampRate]\n           ,[UnitRampRate]\n           ,[TargetTemperature]\n           ,[HoldTimeDuration]\n           ,[Inactive])\n     VALUES (<Values>)\n\n") -> ("error out"=w310:errorcluster, "string out"=w306:string)  [unwired: 8 in]
      n113 = Search and Replace String(replace all?=w303, input string=w306, search string="<A>", replace string=w278, error in=w310) -> (result string=w305:string, error out=w309:errorcluster)  [unwired: 3 in, 2 out]
      n114 = Search and Replace String(replace all?=w303, input string=w305, search string="<B>", replace string=w277, error in=w309) -> (result string=w307:string, error out=w308:errorcluster)  [unwired: 3 in, 2 out]
      n115 = String Subset "Skip 1st ,"(string=w294, offset (0)=1) -> (substring=w296:string)  [unwired: 1 in]
      n116 = Search and Replace String(replace all?=TRUE ("replace all? (F)"), input string=w296, search string="\r\n") -> (result string=w288:string)  [unwired: 5 in, 3 out]
      n117 = Search and Replace String(input string=w307, search string="(<Values>)", replace string=w288, error in=w308) -> (result string=w283:string, error out=w281:errorcluster)  [unwired: 4 in, 2 out]
      n118 = Search and Replace String(replace all?=TRUE ("replace all? (F)"), input string=w283, search string="<C>", replace string=w278, error in=w281) -> (result string=w282:string, error out=w280:errorcluster)  [unwired: 3 in, 2 out]
      n119 = Search and Replace String(replace all?=TRUE ("replace all? (F)"), input string=w282, search string="<D>", replace string=w277, error in=w280) -> (result string=w279:string)  [unwired: 3 in, 3 out]
      n120 = call-poly <vilib>:"DB Tools Execute Query.vi"("error in (no error)"=w316, "SQL query"=w279, "connection reference"=w317) -> ("error out"=w312:errorcluster, "recordset reference"=w313:T18)  [unwired: 5 in]
      n121 = call-poly <vilib>:"DB Tools Free Object.vi"("error in (no error)"=w312, "recordset reference"=w313) -> ("error out"=w314:errorcluster, "connection reference"=w315:T12)  [unwired: 8 in]
    }
    frame "UPDATE [TransactionResult]" {
      n122 = Unbundle By Name(w336) -> ("TransactionNo"=w338:string, "TransactionRunNo"=w337:string)
      n123 = flat-sequence {
        tunnel: [w361] -> w340
        tunnel: w339 -> [w360]
        tunnel: w335 -> [w359]
        frame #0 {
          # "UPDATE ... SET <Values> WHERE ...\nUsed in \nDB - [Execute].[Transaction]\nDB - [Execute].[ActiveProcess]"
          n124 = for {
            tunnel: w360 -> [w370] mode=indexing
            tunnel: w359 -> [w374] mode=indexing
            shift-right: [w371] -> w366
            shift-left: "" -> [w373]
            n125 = Format Into String(w370) -> (resulting string=w369:string)  [unwired: 3 in, 1 out]
            n126 = Search and Replace String(input string=",<A> = '<B>' ", search string="<A>", replace string=w369) -> (result string=w376:string)  [unwired: 5 in, 3 out]
            n127 = Search and Replace String(input string=w376, search string="<B>", replace string=w374) -> (result string=w372:string)  [unwired: 5 in, 3 out]
            n128 = Concatenate Strings(w373, w372) -> (w371:string)
          }
          n129 = Search/Split String "Skip 1st ,"(string=w366, offset (0)=1) -> (match + rest of string=w365:string)  [unwired: 1 in, 2 out]
          n130 = Search and Replace String(replace all?=TRUE ("replace all? (F)"), input string=w365, search string="'NULL'", replace string="NULL" ("replace string (\"\")")) -> (result string=w361:string)  [unwired: 4 in, 3 out]
        }
      }
      n131 = call "DB - Replace DB.Schema.Table.vi"("DB.Schema.Table"=w357, "string in"="USE [<DB>]\n\nUPDATE [<Schema>].[<Table>]\n   SET <Values>\nWHERE [TransactionNo] = '<A>' AND\n[TransactionRunNo] = '<B>' AND\n[Inactive] = '0' \n\n") -> ("error out"=w355:errorcluster, "string out"=w356:string)  [unwired: 8 in]
      n132 = Search and Replace String(input string=w356, search string="<Values>", replace string=w340, error in=w355) -> (result string=w346:string, error out=w344:errorcluster)  [unwired: 4 in, 2 out]
      n133 = Search and Replace String(input string=w346, search string="<A>", replace string=w338, error in=w344) -> (result string=w345:string, error out=w347:errorcluster)  [unwired: 4 in, 2 out]
      n134 = Search and Replace String(input string=w345, search string="<B>", replace string=w337, error in=w347) -> (result string=w341:string)  [unwired: 4 in, 3 out]
      n135 = call-poly <vilib>:"DB Tools Execute Query.vi"("error in (no error)"=w352, "SQL query"=w341, "connection reference"=w353) -> ("error out"=w348:errorcluster, "recordset reference"=w349:T18)  [unwired: 5 in]
      n136 = call-poly <vilib>:"DB Tools Free Object.vi"("error in (no error)"=w348, "recordset reference"=w349) -> ("error out"=w350:errorcluster, "connection reference"=w351:T12)  [unwired: 8 in]
    }
    frame "UPDATE FILESTREAM" {
      n137 = Unbundle By Name(w381) -> ("TransactionNo"=w383:string, "TransactionRunNo"=w382:string)
      n138 = call "DB - Replace DB.Schema.Table.vi"("DB.Schema.Table"=w400, "string in"="USE [<DB>]\n\nUPDATE [<Schema>].[<Table>] \nSET [RawDataFile] = CAST('<R>' as varbinary(max))\n\nWHERE [TransactionNo] = '<A>' AND\n[TransactionRunNo] = '<B>' AND\n[Inactive] = '0' \n\n") -> ("error out"=w398:errorcluster, "string out"=w399:string)  [unwired: 8 in]
      n139 = Search and Replace String(input string=w399, search string="<R>", replace string="String ([RawDataFile] Filestream)", error in=w398) -> (result string=w389:string, error out=w387:errorcluster)  [unwired: 4 in, 2 out]
      n140 = Search and Replace String(input string=w389, search string="<A>", replace string=w383, error in=w387) -> (result string=w388:string, error out=w390:errorcluster)  [unwired: 4 in, 2 out]
      n141 = Search and Replace String(input string=w388, search string="<B>", replace string=w382, error in=w390) -> (result string=w384:string)  [unwired: 4 in, 3 out]
      n142 = call-poly <vilib>:"DB Tools Execute Query.vi"("error in (no error)"=w395, "SQL query"=w384, "connection reference"=w396) -> ("error out"=w391:errorcluster, "recordset reference"=w392:T18)  [unwired: 5 in]
      n143 = call-poly <vilib>:"DB Tools Free Object.vi"("error in (no error)"=w391, "recordset reference"=w392) -> ("error out"=w393:errorcluster, "connection reference"=w394:T12)  [unwired: 8 in]
    }
    frame "SELECT [TransactionResult]" {
      w401 = T5[] [enum."[StartRecordTime]", enum."[MaxRecordedTempTime]", enum."[MinRecordedTempTime]", enum."[EndRecordTime]", enum."[StartHoldTime]", enum."[HoldTimeMaxTempTime]", enum."[HoldTimeMinTempTime]", enum."[EndHoldTime]", enum."[PerformedOn]", enum."[SavedOn]"] items=["[StartRecordTime]", "[StartRecordTemp]", "[MaxRecordedTemp]", "[MaxRecordedTempTime]", "[MinRecordedTemp]", "[MinRecordedTempTime]", "[EndRecordTemp]", "[EndRecordTime]", "[RecordedMinutes]", "[StartHoldTime]", "[StartHoldTemp]", "[HoldTimeMaxTemp]", "[HoldTimeMaxTempTime]", "[HoldTimeMinTemp]", "[HoldTimeMinTempTime]", "[EndHoldTime]", "[EndHoldTemp]", "[HoldDurationMinutes]", "[TempDiffDuringHold]", "[UnitOfTemperature]", "[PerformedBy]", "[PerformedOn]", "[IsTempWithinTol]", "[IsTimeWithinTol]", "[HoldTimePercentage]", "[ProcessStatus]", "[OverallStatus]", "[SequenceStatus]", "[Parameter1]", "[Parameter2]", "[Parameter3]", "[Parameter4]", "[Parameter5]", "[Parameter6]", "[Parameter7]", "[Parameter8]", "[Parameter9]", "[Parameter10]", "[Parameter11]", "[Parameter12]", "[Result]", "[RawDataFile]", "[RawDataFilePath]", "[RawDataFileName]", "[OutputSetId]", "[SavedBy]", "[SavedOn]", "[Inactive]"]
      n144 = Unbundle By Name(w405) -> ("TransactionNo"=w407:string, "TransactionRunNo"=w406:string)
      n145 = for {
        tunnel: w430 -> [w431] mode=indexing
        tunnel: [w432] -> w411 mode=indexing
        tunnel: w401 -> [w434]
        n146 = Search 1D Array(1D array=w434, element=w431) -> (index of element=w433:i32)  [unwired: 1 in]
        n147 = case shown="0, Default" w433 {
          tunnel: w431 -> [w436 _]
          tunnel: [w435 w439] -> w432
          tunnel: w431 -> [_ w440]
          frame 0, Default {
            n148 = Format Into String(format string="FORMAT(%s, 'yyyy-MM-dd HH:mm:ss')", initial string="", w436) -> (resulting string=w435:string)  [unwired: 1 in, 1 out]
          }
          frame -1 {
            n149 = Format Into String(w440) -> (resulting string=w439:string)  [unwired: 3 in, 1 out]
          }
        }
      }
      n150 = Array To Spreadsheet String(delimiter (Tab)=",", array=w411, 3:"" ("format string")) -> (spreadsheet string=w410:string)
      n151 = call "DB - Replace DB.Schema.Table.vi"("DB.Schema.Table"=w428, "string in"="USE [<DB>]\nSELECT <A> FROM\n[<Schema>].[<Table>]\nWHERE [TransactionNo] = '<B>' AND\n[TransactionRunNo] = '<C>' AND\n[Inactive] = '0' ") -> ("string out"=w427:string)  [unwired: 8 in, 1 out]
      n152 = Search and Replace String(input string=w427, search string="<A>", replace string=w410) -> (result string=w425:string)  [unwired: 5 in, 3 out]
      n153 = Search and Replace String(input string=w425, search string="<B>", replace string=w407) -> (result string=w423:string)  [unwired: 5 in, 3 out]
      n154 = Search and Replace String(input string=w423, search string="<C>", replace string=w406) -> (result string=w412:string)  [unwired: 5 in, 3 out]
      n155 = call-poly <vilib>:"DB Tools Execute Query.vi"("SQL query"=w412, "connection reference"=w421) -> ("error out"=w418:errorcluster, "recordset reference"=w420:T18)  [unwired: 6 in]
      n156 = call-poly <vilib>:"DB Tools Fetch Recordset Data.vi"("error in (no error)"=w418, "recordset reference"=w420) -> ("error out"=w417:errorcluster, "recordset data"=w416:variant[][], "recordset reference out"=w419:T18)  [unwired: 3 in]
      n157 = Variant To Data(type=string[][] [], Variant=w416) -> (data=w404:string[][])  [unwired: 1 in, 1 out]
      n158 = call-poly <vilib>:"DB Tools Free Object.vi"("error in (no error)"=w417, "recordset reference"=w419) -> ("error out"=w414:errorcluster, "connection reference"=w413:T12)  [unwired: 8 in]
      n159 = Index Array "Only 1D Result since we are Querying with BOTH Primary Keys"(array=w404, index (row)=0) -> (element=w402:string[])  [unwired: 1 in]
    }
    frame "SELECT [TransactionNo],[TransactionRunNo]" {
      w444 = 1  # [TransactionRunNo]
      w445 = 0  # [TransactionNo]
      # "Called by:\n{Generate Report}"
      n160 = call "DB - Replace DB.Schema.Table.vi"("DB.Schema.Table"=w462, "string in"="USE [<DB>]\nSELECT TOP 1 [TransactionNo],[TransactionRunNo] FROM\n[<Schema>].[<Table>]\nWHERE [RawDataFileName] = '<A>' AND\n[Inactive] = '0' ") -> ("string out"=w461:string)  [unwired: 8 in, 1 out]
      n161 = Search and Replace String(input string=w461, search string="<A>", replace string="[RawDataFileName]") -> (result string=w449:string)  [unwired: 5 in, 3 out]
      n162 = call-poly <vilib>:"DB Tools Execute Query.vi"("SQL query"=w449, "connection reference"=w459) -> ("error out"=w456:errorcluster, "recordset reference"=w458:T18)  [unwired: 6 in]
      n163 = call-poly <vilib>:"DB Tools Fetch Recordset Data.vi"("error in (no error)"=w456, "recordset reference"=w458) -> ("error out"=w455:errorcluster, "recordset data"=w454:variant[][], "recordset reference out"=w457:T18)  [unwired: 3 in]
      n164 = Variant To Data(type=string[][] [], Variant=w454) -> (data=w448:string[][])  [unwired: 1 in, 1 out]
      n165 = call-poly <vilib>:"DB Tools Free Object.vi"("error in (no error)"=w455, "recordset reference"=w457) -> ("error out"=w452:errorcluster, "connection reference"=w451:T12)  [unwired: 8 in]
      n166 = Index Array(array=w448, index (row)=0) -> (element=w446:string[])  [unwired: 1 in]
      n167 = Index Array(array=w446, index #1=w445, index #2=w444) -> (element #1=w442:string, element #2=w441:string)
      n168 = Bundle(w442, w441) -> (w443:cluster{string, string})  [unwired: 1 in]
    }
  }
  "SUMMARY" <- w10
  "connection reference" <- w42
  "SQL 2" <- w14
  "SQL 1" <- w15
  "Transaction" <- w12
  "1D Results" <- w8
  n169 = flat-sequence {
    tunnel: [w464] -> w46
    frame #0 {
      n170 = Tick Count (ms)() -> (millisecond timer value=w464:u32)
    }
  }
  n171 = flat-sequence {
    tunnel: w46 -> [w466]
    frame #0 {
      n172 = Tick Count (ms)() -> (millisecond timer value=w467:u32)
      n173 = Subtract(x=w467, y=w466) -> (x-y=→"ms":u32)
    }
  }
  n174 = case shown="True" w39 {
    tunnel: w10 -> [_ w469]
    tunnel: w42 -> [_ w470]
    frame False {
    }
    frame True {
      n175 = call <vilib>:"DB Tools Close Connection.vi"("error in (no error)"=w469, "connection reference"=w470) -> ("error out"=→"Close error out":errorcluster)  [unwired: 5 in]
    }
  }
  n176 = global write "Global SRTRS.vi" "DB Error"(w10) -> ()
